vi "plcHMI_rev4.vi"() -> ()   [LabVIEW 2020]
doc: "ADS continuos synchronous write example using base blocks. \n\nThe client writes data synchronously and does wait for the respose from server."
uses:
  Agilent/AgilentTotalCluster.ctl
  Agilent/AgilentControl.ctl
  Agilent/Channel Config.ctl
  <vilib>/Platform/TimedLoop/XDataNode/timing_clust.ctl
  <vilib>/Platform/TimedLoop/XDataNode/nitl_modes.ctl
  <vilib>/Platform/TimedLoop/XDataNode/wakeup.ctl
  <userlib>/Beckhoff-LabVIEW-Interface/_DependsOn/With TypeResolving/Write Sync Single TypeResolved.vi
  <userlib>/Beckhoff-LabVIEW-Interface/_DependsOn/With TypeResolving/Read Sync Single TypeResolved.vi
  <vilib>/Platform/TimedLoop/XDataNode/XDataNode.xnode
  <vilib>/Platform/TimedLoop/XDataNode/XDNodeRunTimeDep.lvlib
panel:
  in  "Tab Control":T1(tab)
  out "error out":errorcluster
  in  "Symbol file path - MUST BE ENTERED\nLoad \"ADS Write AND Read Symbols REV X.X.xml\"":path
  out "bHasMached":bool
  out "Write Status":bool
  out "Read Status":bool
  in  "EXIT HMI":bool caption="STOP HMI\nEXIT HMI"
  out "Internal TwinCAT Handle ID Maps":dbl format="%#_12g"
  in  "802L TDK PSU Voltage Rating (abs(Volts))":i32=12000 min=1 max=50000
  in  "802L TDL PSU Peak Power (J/s)":i32=9000 min=1 max=50000
  in  "HVPS Model":u16(ring) items=["802L-12kV,9000J/s", "802L+50kV,9000J/s", "Other"]
  out "Test Interval Fault":bool
  in  "Cycle Time (Sec)":i32=15 min=0
  in  "Voltage Held by PSU":bool
  in  "Log Capacitor Voltage":bool
  in  "Log Temperature Data":bool
  out "Time Since Last Shot":string caption="Elapsed Time Text"
  in  "Duty Cycle":dbl
  in  "Current Control":bool
  out "Expected Voltage":i16
  in  "Dump":bool
  out "EOC":bool
  out "Maximum Test Number Reached":bool
  out "SCR Ready":bool
  in  "START":bool
  in  "STOP":bool
  in  "Hold":bool
  in  "Charge":bool
  in  "Shot":bool
  in  "HV Switch Mode":bool
  in  "CLEAR FAULT":bool
  in  "Manual/Auto":bool=TRUE
  out "Test Interval (Sec)":i32=15 min=0
  in  "Capacitance (uF)":sgl=1e-13 min=0 max=10000 format="%#_6f"
  in  "Target Charge Volt (V) - Min 1500V - TEMPORARY LIMIT 12kV":i32 min=-12000 max=12000 step=1
  out "Estimated Charge Time (seconds)":sgl
  in  "Hold Time Before Shot (seconds)":sgl max=1000
  in  "Max Number of Shots (Test intervals)":i16=1 min=1
  out "Shot Number":i16
  out "Charge Fault":bool=TRUE
  out "Discharge Fault":bool=TRUE
  out "Hold Fault":bool=TRUE
  out "Cap 1 Temp\nExceeded Fault":bool=TRUE
  out "Ambient Temp\nExceeded Fault":bool=TRUE
  out "PSU Fault":bool=TRUE
  out "Control Sys Fault":bool=TRUE
  out "test Running":bool
  out "Test State":string
  out "Cap 1 Voltage":i16
  out "Cap 1 Temperature":i16
  in  "Capacitor Voltage Data Log File Path (.xlsx)":path
  out "Load Temperature":i16
  out "Soft Dump Temp":i16
  out "Ambient Temp":i16
  out "Waveform Chart - Capacitor Voltage (Probe, abs(Volts))":dbl(graph)
  in  "Manual Charge Time (seconds)":sgl max=90
  in  "Reset Test Number":bool
  in  "Cap 1 Fault Temp (Cel)":i16 min=0 max=125
  in  "Capacitor Temperature Data Log File Path (.xlsx)":path
  out "Cap 1 Voltage (HVPS)":i16
  out "Capacitor Voltage":cluster{dbl, dbl}(graph)
  out "EOC":i16(graph)
  out "Soft Exception":bool
  out "PSU HV FB Fault":bool
  out "Charge FB Fault":bool
  out "Softdump FB Fault":bool
  out "SCR FB":i16(graph)
  in  "CH4 Vertical Units":string(combo)="V"
  in  "CH4 Vertical Units/div":dbl=2.0
  in  "Toggle Scope Scale":bool
  in  "CH1 Vertical Units/div":dbl=2.0
  in  "CH1 Vertical Units":string(combo)="V"
  in  "Horizontal Units":enum16{"us", "ms", "s"}(ring)
  in  "Horizontal Units/div":dbl=200.0
  out "Download":bool
  in  "Single":bool
  in  "Stop":bool
  out "Scope Trig":bool
  in  "Agilent Array":T2[](array[typedef])
  out "Process Step":u8
  out "Stop Loops":bool
  # "CONFIGURATION"
  # "Press STOP HMI instead of\nLabView Abort Execution"
  # "PSU V Rating, Peak Power\nactive when OTHER\nis selected"
  # "INPUT VARIABLES - For TDK Lambda 802L\nMust be written to before START"
  # "FAULT STATUSES"
  # "Set to -1 for automated\nfull charge to setpoint"
  # "MANUAL CONTROLS"
  # "Does not record during \"wait\" and appends to data file. Must be named with .xlsx"
  # "HV Switch Configuration"
  # "Records during \"Test Running.\" Must be named with .xlsx"
  # "Control Sys Faults"
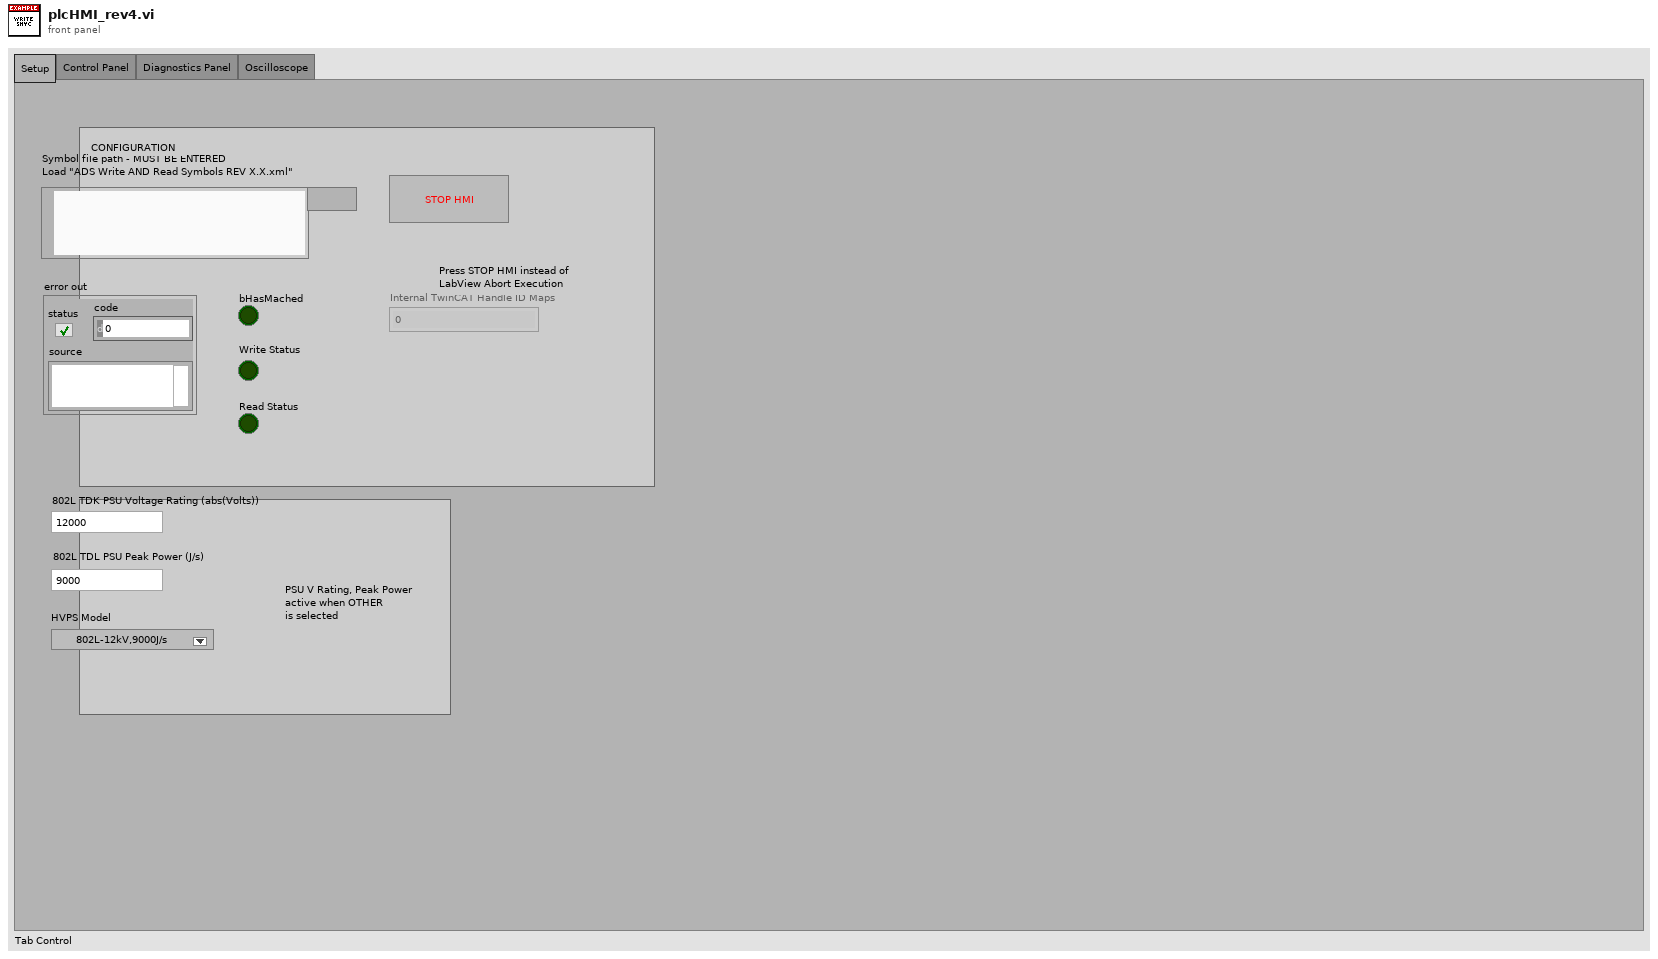
[diagram p1: front panel]
types:
  T1 = enum32{"Setup", "Control Panel", "Diagnostics Panel", "Oscilloscope"}
  T2 = typedef "AgilentTotalCluster.ctl" = cluster{"Agilent Graph":waveform(dbl)[], "Agilent Control":T3, "Agilent Setup Error":errorcluster, "Agilent Present":bool, "Enabled":bool}
  T3 = typedef "AgilentControl.ctl" = cluster{"Trig?":bool, "VISA session":refnum<visa-resource-name>, "Setup to Load":string, "Timeout (ms)":u32, "Desired Samp":enum32{"100", "250", "500", "1000", "2000", "5000", "10000", "20000", "50000", "100000", "200000", "500000", "1000000", "2000000", "4000000", "8000000"}, "Captured Samp":i32, "Desired Channels":T4[]}
  T4 = typedef "Channel Config.ctl" = cluster{"Chan Index":enum16{"Channel1", "Channel2", "Channel3", "Channel4", "MATH"}, "Name":string, "Samples":i32}
  T5 = typedef "XDNodeRunTimeDep.lvlib/timing_clust.ctl" = cluster{"Expected End [f-1]":u64, "Actual End [f-1]":u64, "Finished Late? [f-1]":bool, "Expected End [i-1]":u64, "Actual End [i-1]":u64, "Finished Late? [i-1]":bool, "Expected Start [i]":u64, "Actual Start [i]":u64, "Expected Start [f]":u64, "Actual Start [f]":u64, "Source Name":string, "Structure Name":string, "Period":i64, "Deadline":i64, "Offset":i64, "Start":i64, "Priority":i32, "Timeout":i32, "Mode":T6, "Wakeup Reason":T7, "Error":errorcluster, "Source Type":string, "Secondary Source Type":string, "Global End Time":u64, "Global Start Time":u64, "Frame Duration":u64, "Iteration Duration":u64, "Assigned CPU":i32, "I/O Scan Engine Mode":u32}
  T6 = typedef "XDNodeRunTimeDep.lvlib/nitl_modes.ctl" = enum32{"No Change", "Process missed periods, maintain original phase", "Discard missed periods, maintain original phase", "Process missed periods, ignore original phase", "Discard missed periods, ignore original phase"}
  T7 = typedef "XDNodeRunTimeDep.lvlib/wakeup.ctl" = enum32{"Normal", "Aborted", "Asynchronous wakeup", "Timing source error", "Timed loop error", "Timeout"}
  T8 = cluster{"Agilent Array[0]":T2, "Agilent Array[1]":T2, "Agilent Array[2]":T2, "Agilent Array[3]":T2, "Agilent Array[4]":T2, "Agilent Array[5]":T2, "Agilent Array[6]":T2, "Agilent Array[7]":T2, "Agilent Array[8]":T2}
  T9 = enum32{"100", "250", "500", "1000", "2000", "5000", "10000", "20000", "50000", "100000", "200000", "500000", "1000000", "2000000", "4000000", "8000000"}
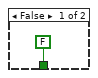
[diagram p2: hidden frame]
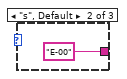
[diagram p5: hidden frame]
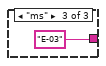
[diagram p6: hidden frame]
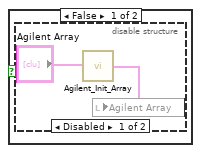
[diagram p7: hidden frame]
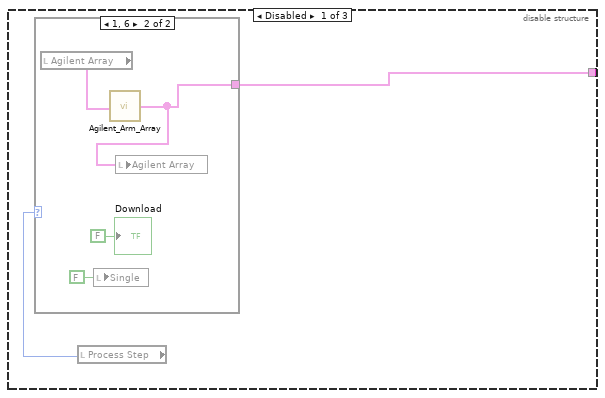
[diagram p11: hidden frame]
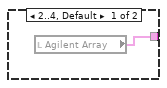
[diagram p12: hidden frame]
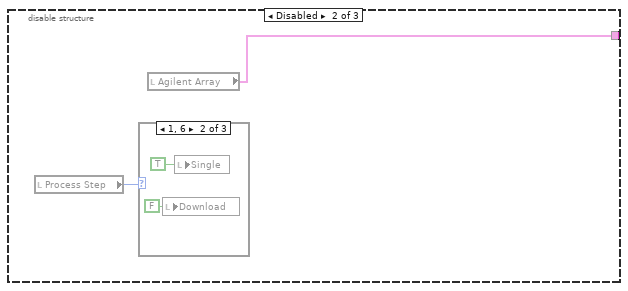
[diagram p13: hidden frame]
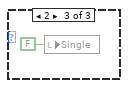
[diagram p15: hidden frame]
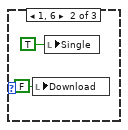
[diagram p17: hidden frame]
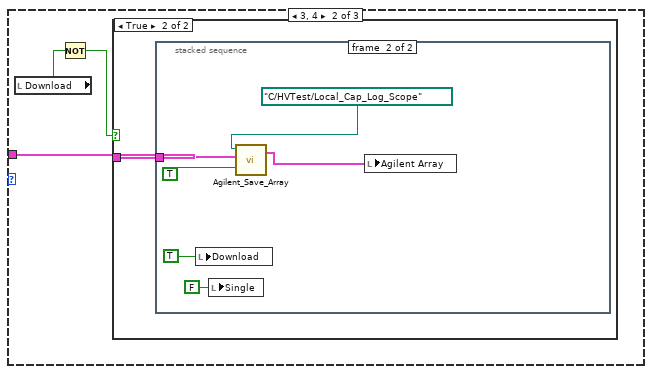
[diagram p19: hidden frame]
diagram:
  w88 = u16 17 items=["SyncLatest"=17, "AsyncLatest"=33] ("WriterMode")
  w158 = u16 33 items=["SyncLatest"=17, "AsyncLatest"=33] ("WriterMode")
  w198 = u16 33 items=["SyncLatest"=17, "AsyncLatest"=33] ("WriterMode")
  w217 = u16 33 items=["SyncLatest"=17, "AsyncLatest"=33] ("WriterMode")
  w236 = u16 33 items=["SyncLatest"=17, "AsyncLatest"=33] ("WriterMode")
  w255 = u16 33 items=["SyncLatest"=17, "AsyncLatest"=33] ("WriterMode")
  w274 = u16 33 items=["SyncLatest"=17, "AsyncLatest"=33] ("WriterMode")
  w293 = u16 17 items=["SyncLatest"=17, "AsyncLatest"=33] ("WriterMode")
  w312 = u16 17 items=["SyncLatest"=17, "AsyncLatest"=33] ("WriterMode")
  w331 = u16 17 items=["SyncLatest"=17, "AsyncLatest"=33] ("WriterMode")
  w350 = u16 17 items=["SyncLatest"=17, "AsyncLatest"=33] ("WriterMode")
  w369 = u16 17 items=["SyncLatest"=17, "AsyncLatest"=33] ("WriterMode")
  w388 = u16 17 items=["SyncLatest"=17, "AsyncLatest"=33] ("WriterMode")
  w407 = u16 17 items=["SyncLatest"=17, "AsyncLatest"=33] ("WriterMode")
  w422 = u16 17 items=["SyncLatest"=17, "AsyncLatest"=33] ("WriterMode")
  # "Variables/ Control"
  # "Documentation:\nCode separated vertically into two main sections - Write and read\nThey are further separated into BOOL and numeric\nThe OR gates wire all the error lines and the EXIT HMI button to a WHILE LOOP STOP\nThere current delay time on the routine is 100ms\nAll the AND gates connect the typecast resolve lines to the bHasMatched indicator\nThe second and third set of AND gates connect the write statuses to the Write Status indicator\nThe same is done for the read status indicator"
  # "WRITE NUMERICS"
  # "WRITE BOOLS"
  # "Select Symbol N"
  # "Read Initialization"
  # "Release \nTypeResolver"
  # "Release Writer"
  # "Send Request"
  # "Init \nTypeResolver"
  # "Init Writer"
  # "Select Symbol"
  # "Initialization"
  # "Call Release handle block\nat the end, when all nodes\nhave finished their execution"
  # "There must be only one release\nafter every init block.\nRelease block must be called\nalways at the end."
  # "Release"
  # "Symbol Interface"
  n1 = disable-structure shown="Enabled" {
    disable-tunnel: [w428 _] -> w426
    disable-tunnel: [w427 w430] -> w425
    frame Disabled {
      # "Using Symbol Interface"
      n2 = call <userlib>:"Symbol Interface.vi"() -> ("PortInfo"=w427:string, "error out"=w428:errorcluster)  [unwired: 14 in]
    }
    frame Enabled {
      # "Using Symbol File"
      n3 = Path To String(path="Symbol file path - MUST BE ENTERED\nLoad \"ADS Write AND Read Symbols REV X.X.xml\"") -> (string=w430:string)
    }
  }
  n4 = call <userlib>:"Init.vi"("XMLDescription"=w425, "error in (no error)"=w426) -> ("Handle"=w38:u32, "ReadGrpSymbols"=w20:string[], "WriteGrpSymbols"=w26:string[], "error out"=w2:errorcluster)  [unwired: 9 in, 1 out]
  n5 = Index Array(array=w26, index=0) -> (element=w13:string)
  n6 = Index Array(array=w26, index=21) -> (element=w25:string)
  n7 = Index Array(array=w26, index=20) -> (element=w31:string)
  n8 = Index Array(array=w26, index=14) -> (element=w3:string)
  n9 = Index Array(array=w26, index=9) -> (element=w275:string)
  n10 = Index Array(array=w26, index=10) -> (element=w256:string)
  n11 = Index Array(array=w26, index=12) -> (element=w218:string)
  n12 = Index Array(array=w26, index=11) -> (element=w237:string)
  n13 = Index Array(array=w26, index=13) -> (element=w199:string)
  n14 = Index Array(array=w26, index=18) -> (element=w39:string)
  n15 = Index Array(array=w26, index=19) -> (element=w32:string)
  n16 = Index Array(array=w26, index=7) -> (element=w294:string)
  n17 = Index Array(array=w26, index=2) -> (element=w389:string)
  n18 = Index Array(array=w26, index=3) -> (element=w370:string)
  n19 = Index Array(array=w26, index=5) -> (element=w332:string)
  n20 = Index Array(array=w26, index=4) -> (element=w351:string)
  n21 = Index Array(array=w26, index=6) -> (element=w313:string)
  n22 = Index Array(array=w26, index=1) -> (element=w408:string)
  n23 = Index Array(array=w26, index=16) -> (element=w6:string)
  n24 = Index Array(array=w26, index=8) -> (element=w87:string)
  n25 = Index Array(array=w26, index=15) -> (element=w159:string)
  n26 = Index Array(array=w26, index=17) -> (element=w8:string)
  n27 = call <userlib>:"Init Writer.vi"("Handle"=w38, "SymbolName"=w275, "WriterMode"=w274, "error constant"=w2) -> ("Handle"=w270:u32, "SymbolName"=w269:string, "WriterMode"=w268:u16, "WriteHandle"=w266:u32, "error IO"=w267:errorcluster)  [unwired: 7 in]
  n28 = call <userlib>:"Init Writer.vi"("Handle"=w38, "SymbolName"=w256, "WriterMode"=w255, "error constant"=w2) -> ("Handle"=w254:u32, "SymbolName"=w253:string, "WriterMode"=w252:u16, "WriteHandle"=w251:u32, "error IO"=w250:errorcluster)  [unwired: 7 in]
  n29 = call <userlib>:"Init Writer.vi"("Handle"=w38, "SymbolName"=w218, "WriterMode"=w217, "error constant"=w2) -> ("Handle"=w216:u32, "SymbolName"=w215:string, "WriterMode"=w214:u16, "WriteHandle"=w213:u32, "error IO"=w212:errorcluster)  [unwired: 7 in]
  n30 = call <userlib>:"Init Type.vi"("Handle"=w38, "SymbolName"=w275, "error in"=w2) -> ("Handle"=w259:u32, "TypeHdl"=w258:u32, "error IO"=w257:errorcluster)  [unwired: 7 in, 3 out]
  n31 = call <userlib>:"Init Type.vi"("Handle"=w38, "SymbolName"=w256, "error in"=w2) -> ("Handle"=w249:u32, "TypeHdl"=w248:u32, "error IO"=w247:errorcluster)  [unwired: 7 in, 3 out]
  n32 = call <userlib>:"Init Writer.vi"("Handle"=w38, "SymbolName"=w237, "WriterMode"=w236, "error constant"=w2) -> ("Handle"=w235:u32, "SymbolName"=w234:string, "WriterMode"=w233:u16, "WriteHandle"=w232:u32, "error IO"=w231:errorcluster)  [unwired: 7 in]
  n33 = call <userlib>:"Init Type.vi"("Handle"=w38, "SymbolName"=w218, "error in"=w2) -> ("Handle"=w211:u32, "TypeHdl"=w210:u32, "error IO"=w209:errorcluster)  [unwired: 7 in, 3 out]
  n34 = call <userlib>:"Init Writer.vi"("Handle"=w38, "SymbolName"=w199, "WriterMode"=w198, "error constant"=w2) -> ("Handle"=w197:u32, "SymbolName"=w196:string, "WriterMode"=w195:u16, "WriteHandle"=w194:u32, "error IO"=w193:errorcluster)  [unwired: 7 in]
  n35 = call <userlib>:"Init Type.vi"("Handle"=w38, "SymbolName"=w237, "error in"=w2) -> ("Handle"=w230:u32, "TypeHdl"=w229:u32, "error IO"=w228:errorcluster)  [unwired: 7 in, 3 out]
  n36 = call <userlib>:"Init Type.vi"("Handle"=w38, "SymbolName"=w199, "error in"=w2) -> ("Handle"=w192:u32, "TypeHdl"=w191:u32, "error IO"=w190:errorcluster)  [unwired: 7 in, 3 out]
  n37 = call <userlib>:"Init Writer.vi"("Handle"=w38, "SymbolName"=w294, "WriterMode"=w293, "error constant"=w2) -> ("Handle"=w292:u32, "SymbolName"=w291:string, "WriterMode"=w290:u16, "WriteHandle"=w289:u32, "error IO"=w288:errorcluster)  [unwired: 7 in]
  n38 = call <userlib>:"Init Writer.vi"("Handle"=w38, "SymbolName"=w389, "WriterMode"=w388, "error constant"=w2) -> ("Handle"=w384:u32, "SymbolName"=w383:string, "WriterMode"=w382:u16, "WriteHandle"=w380:u32, "error IO"=w381:errorcluster)  [unwired: 7 in]
  n39 = call <userlib>:"Init Writer.vi"("Handle"=w38, "SymbolName"=w370, "WriterMode"=w369, "error constant"=w2) -> ("Handle"=w368:u32, "SymbolName"=w367:string, "WriterMode"=w366:u16, "WriteHandle"=w365:u32, "error IO"=w364:errorcluster)  [unwired: 7 in]
  n40 = call <userlib>:"Init Writer.vi"("Handle"=w38, "SymbolName"=w332, "WriterMode"=w331, "error constant"=w2) -> ("Handle"=w330:u32, "SymbolName"=w329:string, "WriterMode"=w328:u16, "WriteHandle"=w327:u32, "error IO"=w326:errorcluster)  [unwired: 7 in]
  n41 = call <userlib>:"Init Type.vi"("Handle"=w38, "SymbolName"=w294, "error in"=w2) -> ("Handle"=w287:u32, "TypeHdl"=w286:u32, "error IO"=w285:errorcluster)  [unwired: 7 in, 3 out]
  n42 = call <userlib>:"Init Type.vi"("Handle"=w38, "SymbolName"=w389, "error in"=w2) -> ("Handle"=w373:u32, "TypeHdl"=w372:u32, "error IO"=w371:errorcluster)  [unwired: 7 in, 3 out]
  n43 = call <userlib>:"Init Type.vi"("Handle"=w38, "SymbolName"=w370, "error in"=w2) -> ("Handle"=w363:u32, "TypeHdl"=w362:u32, "error IO"=w361:errorcluster)  [unwired: 7 in, 3 out]
  n44 = call <userlib>:"Init Writer.vi"("Handle"=w38, "SymbolName"=w351, "WriterMode"=w350, "error constant"=w2) -> ("Handle"=w349:u32, "SymbolName"=w348:string, "WriterMode"=w347:u16, "WriteHandle"=w346:u32, "error IO"=w345:errorcluster)  [unwired: 7 in]
  n45 = call <userlib>:"Init Type.vi"("Handle"=w38, "SymbolName"=w332, "error in"=w2) -> ("Handle"=w325:u32, "TypeHdl"=w324:u32, "error IO"=w323:errorcluster)  [unwired: 7 in, 3 out]
  n46 = call <userlib>:"Init Writer.vi"("Handle"=w38, "SymbolName"=w313, "WriterMode"=w312, "error constant"=w2) -> ("Handle"=w311:u32, "SymbolName"=w310:string, "WriterMode"=w309:u16, "WriteHandle"=w308:u32, "error IO"=w307:errorcluster)  [unwired: 7 in]
  n47 = call <userlib>:"Init Type.vi"("Handle"=w38, "SymbolName"=w351, "error in"=w2) -> ("Handle"=w344:u32, "TypeHdl"=w343:u32, "error IO"=w342:errorcluster)  [unwired: 7 in, 3 out]
  n48 = call <userlib>:"Init Type.vi"("Handle"=w38, "SymbolName"=w313, "error in"=w2) -> ("Handle"=w306:u32, "TypeHdl"=w305:u32, "error IO"=w304:errorcluster)  [unwired: 7 in, 3 out]
  n49 = call <userlib>:"Init Writer.vi"("Handle"=w38, "SymbolName"=w408, "WriterMode"=w407, "error constant"=w2) -> ("Handle"=w406:u32, "SymbolName"=w405:string, "WriterMode"=w404:u16, "WriteHandle"=w403:u32, "error IO"=w402:errorcluster)  [unwired: 7 in]
  n50 = call <userlib>:"Init Type.vi"("Handle"=w38, "SymbolName"=w408, "error in"=w2) -> ("Handle"=w401:u32, "TypeHdl"=w400:u32, "error IO"=w399:errorcluster)  [unwired: 7 in, 3 out]
  n51 = call <userlib>:"Init Writer.vi"("Handle"=w38, "SymbolName"=w13, "WriterMode"=w422, "error constant"=w2) -> ("Handle"=w421:u32, "SymbolName"=w420:string, "WriterMode"=w419:u16, "WriteHandle"=w418:u32, "error IO"=w417:errorcluster)  [unwired: 7 in]
  n52 = call <userlib>:"Init Type.vi"("Handle"=w38, "SymbolName"=w13, "error in"=w2) -> ("Handle"=w416:u32, "TypeHdl"=w415:u32, "error IO"=w410:errorcluster)  [unwired: 7 in, 3 out]
  n53 = call <userlib>:"Init Writer.vi"("Handle"=w38, "SymbolName"=w159, "WriterMode"=w158, "error constant"=w2) -> ("Handle"=w154:u32, "SymbolName"=w153:string, "WriterMode"=w152:u16, "WriteHandle"=w144:u32, "error IO"=w151:errorcluster)  [unwired: 7 in]
  n54 = call <userlib>:"Init Type.vi"("Handle"=w38, "SymbolName"=w159, "error in"=w2) -> ("Handle"=w149:u32, "TypeHdl"=w147:u32, "error IO"=w148:errorcluster)  [unwired: 7 in, 3 out]
  n55 = Index Array(array=w20, index=2) -> (element=w140:string)
  n56 = Index Array(array=w20, index=4) -> (element=w136:string)
  n57 = call <userlib>:"Init Writer.vi"("Handle"=w38, "SymbolName"=w87, "WriterMode"=w88, "error constant"=w2) -> ("Handle"=w86:u32, "SymbolName"=w85:string, "WriterMode"=w84:u16, "WriteHandle"=w83:u32, "error IO"=w82:errorcluster)  [unwired: 7 in]
  n58 = Index Array(array=w20, index=1) -> (element=w176:string)
  n59 = Index Array(array=w20, index=21) -> (element=w53:string)
  n60 = Index Array(array=w20, index=22) -> (element=w50:string)
  n61 = call <userlib>:"Init Type.vi"("Handle"=w38, "SymbolName"=w87, "error in"=w2) -> ("Handle"=w81:u32, "TypeHdl"=w80:u32, "error IO"=w79:errorcluster)  [unwired: 7 in, 3 out]
  n62 = Index Array(array=w20, index=0) -> (element=w175:string)
  n63 = Index Array(array=w20, index=3) -> (element=w137:string)
  n64 = Index Array(array=w20, index=20) -> (element=w58:string)
  n65 = Index Array(array=w20, index=23) -> (element=w49:string)
  n66 = Index Array(array=w20, index=16) -> (element=w142:string)
  n67 = Index Array(array=w20, index=24) -> (element=w47:string)
  n68 = Index Array(array=w20, index=11) -> (element=w164:string)
  n69 = Index Array(array=w20, index=10) -> (element=w165:string)
  n70 = Index Array(array=w20, index=17) -> (element=w61:string)
  n71 = Index Array(array=w20, index=18) -> (element=w60:string)
  n72 = Index Array(array=w20, index=13) -> (element=w162:string)
  n73 = Index Array(array=w20, index=27) -> (element=w18:string)
  n74 = Index Array(array=w20, index=12) -> (element=w163:string)
  n75 = Index Array(array=w20, index=15) -> (element=w160:string)
  n76 = Index Array(array=w20, index=19) -> (element=w59:string)
  n77 = Index Array(array=w20, index=26) -> (element=w19:string)
  n78 = Index Array(array=w20, index=5) -> (element=w72:string)
  n79 = Index Array(array=w20, index=6) -> (element=w130:string)
  n80 = Index Array(array=w20, index=9) -> (element=w174:string)
  n81 = Index Array(array=w20, index=14) -> (element=w161:string)
  n82 = Index Array(array=w20, index=8) -> (element=w132:string)
  n83 = Index Array(array=w20, index=25) -> (element=w36:string)
  n84 = Index Array(array=w20, index=7) -> (element=w131:string)
  n85 = node-c288(i64 10 ("Period")) -> (w96:T5)  [unwired: 2 in]
  n86 = timed-loop {
    tunnel: w421 -> [w733]
    tunnel: w420 -> [w732]
    tunnel: w419 -> [w731]
    tunnel: w418 -> [w730]
    tunnel: w416 -> [w975]
    tunnel: w415 -> [w974]
    tunnel: [w728] -> w414
    tunnel: [w727] -> w413
    tunnel: [w973] -> w412
    tunnel: [w972] -> w411
    tunnel: w406 -> [w970]
    tunnel: w405 -> [w969]
    tunnel: w404 -> [w968]
    tunnel: w403 -> [w967]
    tunnel: w401 -> [w965]
    tunnel: w400 -> [w964]
    tunnel: [w962] -> w397
    tunnel: [w961] -> w396
    tunnel: [w960] -> w394
    tunnel: [w959] -> w393
    tunnel: w384 -> [w958]
    tunnel: w383 -> [w957]
    tunnel: w382 -> [w956]
    tunnel: w380 -> [w954]
    tunnel: [w953] -> w379
    tunnel: [w952] -> w378
    tunnel: [w951] -> w375
    tunnel: [w950] -> w374
    tunnel: w373 -> [w949]
    tunnel: w372 -> [w948]
    tunnel: w368 -> [w946]
    tunnel: w367 -> [w945]
    tunnel: w366 -> [w944]
    tunnel: w365 -> [w943]
    tunnel: w363 -> [w941]
    tunnel: w362 -> [w940]
    tunnel: [w938] -> w359
    tunnel: [w937] -> w358
    tunnel: [w936] -> w356
    tunnel: [w935] -> w355
    tunnel: w349 -> [w934]
    tunnel: w348 -> [w933]
    tunnel: w347 -> [w932]
    tunnel: w346 -> [w931]
    tunnel: w344 -> [w929]
    tunnel: w343 -> [w928]
    tunnel: [w926] -> w340
    tunnel: [w925] -> w339
    tunnel: [w924] -> w337
    tunnel: [w923] -> w336
    tunnel: w330 -> [w922]
    tunnel: w329 -> [w921]
    tunnel: w328 -> [w920]
    tunnel: w327 -> [w919]
    tunnel: w325 -> [w917]
    tunnel: w324 -> [w916]
    tunnel: [w914] -> w321
    tunnel: [w913] -> w320
    tunnel: [w912] -> w318
    tunnel: [w911] -> w317
    tunnel: w311 -> [w910]
    tunnel: w310 -> [w909]
    tunnel: w309 -> [w908]
    tunnel: w308 -> [w907]
    tunnel: w306 -> [w905]
    tunnel: w305 -> [w904]
    tunnel: [w902] -> w302
    tunnel: [w901] -> w301
    tunnel: [w900] -> w299
    tunnel: [w899] -> w298
    tunnel: w292 -> [w898]
    tunnel: w291 -> [w897]
    tunnel: w290 -> [w896]
    tunnel: w289 -> [w895]
    tunnel: w287 -> [w893]
    tunnel: w286 -> [w892]
    tunnel: [w890] -> w283
    tunnel: [w889] -> w282
    tunnel: [w888] -> w280
    tunnel: [w887] -> w279
    tunnel: w270 -> [w886]
    tunnel: w269 -> [w885]
    tunnel: w268 -> [w884]
    tunnel: w266 -> [w882]
    tunnel: [w881] -> w265
    tunnel: [w880] -> w264
    tunnel: [w879] -> w261
    tunnel: [w878] -> w260
    tunnel: w259 -> [w877]
    tunnel: w258 -> [w876]
    tunnel: w254 -> [w874]
    tunnel: w253 -> [w873]
    tunnel: w252 -> [w872]
    tunnel: w251 -> [w871]
    tunnel: w249 -> [w869]
    tunnel: w248 -> [w868]
    tunnel: [w866] -> w245
    tunnel: [w865] -> w244
    tunnel: [w864] -> w242
    tunnel: [w863] -> w241
    tunnel: w235 -> [w862]
    tunnel: w234 -> [w861]
    tunnel: w233 -> [w860]
    tunnel: w232 -> [w859]
    tunnel: w230 -> [w857]
    tunnel: w229 -> [w856]
    tunnel: [w854] -> w226
    tunnel: [w853] -> w225
    tunnel: [w852] -> w223
    tunnel: [w851] -> w222
    tunnel: w216 -> [w850]
    tunnel: w215 -> [w849]
    tunnel: w214 -> [w848]
    tunnel: w213 -> [w847]
    tunnel: w211 -> [w845]
    tunnel: w210 -> [w844]
    tunnel: [w842] -> w207
    tunnel: [w841] -> w206
    tunnel: [w840] -> w204
    tunnel: [w839] -> w203
    tunnel: w197 -> [w838]
    tunnel: w196 -> [w837]
    tunnel: w195 -> [w836]
    tunnel: w194 -> [w835]
    tunnel: w192 -> [w833]
    tunnel: w191 -> [w832]
    tunnel: [w830] -> w188
    tunnel: [w829] -> w187
    tunnel: [w828] -> w185
    tunnel: [w827] -> w184
    tunnel: w176 -> [w826]
    tunnel: w175 -> [w825]
    tunnel: w174 -> [w824]
    tunnel: [w823] -> w125
    tunnel: w165 -> [w822]
    tunnel: w164 -> [w821]
    tunnel: w163 -> [w820]
    tunnel: w162 -> [w819]
    tunnel: w161 -> [w818]
    tunnel: w160 -> [w817]
    tunnel: [w816] -> w93
    tunnel: [w815] -> w124
    tunnel: [w814] -> w123
    tunnel: [w813] -> w122
    tunnel: [w812] -> w121
    tunnel: [w756] -> w120
    tunnel: [w754] -> w119
    shift-right: [w657] -> w424
    shift-left: w417 -> [w729]
    shift-right: [w656] -> w423
    shift-left: w410 -> [w971]
    shift-right: [w654] -> w395
    shift-left: w402 -> [w966]
    shift-right: [w653] -> w392
    shift-left: w399 -> [w963]
    shift-right: [w651] -> w377
    shift-left: w381 -> [w955]
    shift-right: [w650] -> w376
    shift-left: w371 -> [w947]
    shift-right: [w648] -> w357
    shift-left: w364 -> [w942]
    shift-right: [w647] -> w354
    shift-left: w361 -> [w939]
    shift-right: [w645] -> w338
    shift-left: w345 -> [w930]
    shift-right: [w644] -> w335
    shift-left: w342 -> [w927]
    shift-right: [w642] -> w319
    shift-left: w326 -> [w918]
    shift-right: [w641] -> w316
    shift-left: w323 -> [w915]
    shift-right: [w639] -> w300
    shift-left: w307 -> [w906]
    shift-right: [w638] -> w297
    shift-left: w304 -> [w903]
    shift-right: [w636] -> w281
    shift-left: w288 -> [w894]
    shift-right: [w635] -> w278
    shift-left: w285 -> [w891]
    shift-right: [w634] -> w263
    shift-left: w267 -> [w883]
    shift-right: [w633] -> w262
    shift-left: w257 -> [w875]
    shift-right: [w631] -> w243
    shift-left: w250 -> [w870]
    shift-right: [w630] -> w240
    shift-left: w247 -> [w867]
    shift-right: [w628] -> w224
    shift-left: w231 -> [w858]
    shift-right: [w627] -> w221
    shift-left: w228 -> [w855]
    shift-right: [w625] -> w205
    shift-left: w212 -> [w846]
    shift-right: [w624] -> w202
    shift-left: w209 -> [w843]
    shift-right: [w622] -> w186
    shift-left: w193 -> [w834]
    shift-right: [w621] -> w183
    shift-left: w190 -> [w831]
    tunnel: w154 -> [w796]
    tunnel: w153 -> [w795]
    tunnel: w152 -> [w794]
    tunnel: [w792] -> w12
    tunnel: [w791] -> w150
    tunnel: w149 -> [w790]
    tunnel: w147 -> [w788]
    tunnel: [w787] -> w146
    tunnel: [w786] -> w145
    tunnel: w144 -> [w785]
    tunnel: w142 -> [w784]
    tunnel: [w755] -> w118
    tunnel: [w778] -> w127
    tunnel: w2 -> [w777]
    tunnel: [w775] -> w126
    tunnel: w140 -> [w774]
    tunnel: w137 -> [w770]
    tunnel: w136 -> [w769]
    tunnel: [w760] -> w128
    tunnel: [w759] -> w129
    tunnel: w132 -> [w753]
    tunnel: w131 -> [w752]
    tunnel: w130 -> [w751]
    tunnel: [w738] -> w69
    tunnel: [w737] -> w68
    tunnel: [w736] -> w67
    timing: w96 -> [_]
    timing-out: [_] -> w95
    tunnel: w38 -> [w726]
    tunnel: [w619] -> w71
    tunnel: w86 -> [w614]
    tunnel: w85 -> [w613]
    tunnel: w84 -> [w612]
    tunnel: w83 -> [w611]
    tunnel: w81 -> [w609]
    tunnel: w80 -> [w608]
    tunnel: [w605] -> w78
    tunnel: [w604] -> w77
    tunnel: [w603] -> w76
    tunnel: [w602] -> w75
    tunnel: [w595] -> w70
    tunnel: w72 -> [w591]
    tunnel: [w590] -> w66
    tunnel: w61 -> [w586]
    tunnel: w60 -> [w581]
    tunnel: w59 -> [w580]
    tunnel: w58 -> [w579]
    tunnel: [w576] -> w57
    tunnel: [w574] -> w56
    tunnel: [w569] -> w55
    tunnel: [w568] -> w42
    tunnel: w53 -> [w566]
    tunnel: w50 -> [w541]
    tunnel: w49 -> [w540]
    tunnel: w47 -> [w533]
    tunnel: [w529] -> w46
    tunnel: [w528] -> w45
    tunnel: [w527] -> w44
    tunnel: [w526] -> w43
    tunnel: w39 -> [w525]
    tunnel: w38 -> [w438]
    tunnel: w2 -> [w524]
    tunnel: [w521] -> w30
    tunnel: [w520] -> _
    tunnel: w36 -> [w516]
    tunnel: [w512] -> w35
    tunnel: w32 -> [w511]
    tunnel: w31 -> [w510]
    tunnel: w2 -> [w487]
    tunnel: [w505] -> w29
    tunnel: [w504] -> w28
    tunnel: w25 -> [w491]
    tunnel: [w486] -> w24
    tunnel: w19 -> [w473]
    tunnel: w18 -> [w472]
    tunnel: [w467] -> w17
    tunnel: [w466] -> w16
    shift-right: [w464] -> w15
    shift-left: w151 -> [w793]
    shift-right: [w463] -> w14
    shift-left: w148 -> [w789]
    tunnel: w2 -> [w456]
    tunnel: [w453] -> w7
    shift-right: [w461] -> w10
    shift-left: w82 -> [w610]
    shift-right: [w460] -> w9
    shift-left: w79 -> [w607]
    tunnel: w8 -> [w455]
    tunnel: w6 -> [w448]
    tunnel: w2 -> [w447]
    tunnel: [w446] -> w5
    tunnel: w3 -> [w439]
    tunnel: w2 -> [w437]
    tunnel: [w436] -> w1
    stop <- w431 stop-if-true
    # "Stop Loop on Error (OR gates)"
    # "Error Stop Loop AND"
    # "Typecast Match AND"
    # "Write Status AND"
    # "READ BOOLS"
    # "READ NUMERICS"
    # "STOP HMI via error or EXIT button"
    # "Check Read status and\nthen convert Variant \nto LabVIEW type (AND gates)"
    # "Sync Read Single"
    n87 = node-c288() -> (w620:errorcluster)  [unwired: 1 in]
    n88 = disable-structure shown="Enabled" {
      frame Enabled {
        n89 = flat-sequence {
          tunnel: [w1111] -> w1055
          tunnel: w1055 -> [w1130]
          frame #0 {
            n90 = disable-structure shown="Enabled" {
              frame Enabled {
                n91 = feedback #1(TRUE) -> (w1057:bool)
                n92 = And(x=TRUE, y=w1057) -> (x .and. y?=w1060:bool)
                n93 = case shown="True" w1060 {
                  tunnel: [FALSE FALSE] -> w1058
                  frame False {
                  }
                  frame True {
                    n94 = local read "Agilent Array"() -> (w1063:T2[])
                    n95 = call "Agilent_Init_Array.vi"("Agilent Array In"=w1063) -> ("Agilent Array Out"=w1064:T2[])
                    n96 = call "Agilent_Arm_Array.vi"("Agilent Array In"=w1064) -> ("Agilent Array Out"=w1062:T2[])
                    n97 = local write "Agilent Array"(w1062) -> ()
                  }
                }
                n98 = feedback-in #1(w1058) -> ()
              }
              frame Disabled {
              }
            }
          }
          frame #1 {
            n99 = case shown="True" "Toggle Scope Scale" {
              frame False {
              }
              frame True {
                n100 = Number To Decimal String(number="CH4 Vertical Units/div") -> (decimal integer string=w1070:string)  [unwired: 1 in]
                n101 = Number To Decimal String(number="Horizontal Units/div") -> (decimal integer string=w1078:string)  [unwired: 1 in]
                n102 = Number To Decimal String(number="CH1 Vertical Units/div") -> (decimal integer string=w1076:string)  [unwired: 1 in]
                n103 = case shown="\"us\"" "Horizontal Units" {
                  tunnel: ["E-06" "E-00" "E-03"] -> w1087
                  frame "us" {
                  }
                  frame "s", Default {
                  }
                  frame "ms" {
                  }
                }
                n104 = Concatenate Strings(":CHAN4:SCAL " ("write buffer"), w1070, "CH4 Vertical Units") -> (w1069:string)
                n105 = Concatenate Strings(":CHAN1:SCAL " ("write buffer"), w1076, "CH1 Vertical Units") -> (w1083:string)
                n106 = Concatenate Strings(":TIM:SCAL " ("write buffer"), w1078, w1087) -> (w1086:string)
                n107 = VISA Open(VISA resource name=refnum<visa-resource-name> "HV_Test_Scope") -> (VISA resource name=w1081:refnum<visa-resource-name>, error out=w1082:errorcluster)  [unwired: 4 in]
                n108 = VISA Write(VISA resource name=w1081, write buffer=w1086, error in (no error)=w1082) -> (VISA resource name out=w1090:refnum<visa-resource-name>, error out=w1089:errorcluster)  [unwired: 1 out]
                n109 = VISA Write(VISA resource name=w1090, write buffer=w1083, error in (no error)=w1089) -> (VISA resource name out=w1075:refnum<visa-resource-name>, error out=w1073:errorcluster)  [unwired: 1 out]
                n110 = VISA Write(VISA resource name=w1075, write buffer=w1069, error in (no error)=w1073) -> (VISA resource name out=w1074:refnum<visa-resource-name>, error out=w1072:errorcluster)  [unwired: 1 out]
                n111 = VISA Close(VISA resource name=w1074, error in (no error)=w1072) -> ()  [unwired: 1 out]
              }
            }
          }
          frame #2 {
            n112 = disable-structure shown="Enabled" {
              frame Enabled {
                n113 = case shown="True" "Stop" {
                  frame False {
                    n114 = disable-structure shown="Disabled" {
                      frame Disabled {
                        n115 = call "Agilent_Init_Array.vi"("Agilent Array In"="Agilent Array") -> ("Agilent Array Out"=w1097:T2[])
                        n116 = local write "Agilent Array"(w1097) -> ()
                      }
                      frame Enabled {
                      }
                    }
                  }
                  frame True {
                    n117 = VISA Open(VISA resource name=refnum<visa-resource-name> "HV_Test_Scope") -> (VISA resource name=w1103:refnum<visa-resource-name>, error out=w1104:errorcluster)  [unwired: 4 in]
                    n118 = VISA Write(VISA resource name=w1103, write buffer=":STOP", error in (no error)=w1104) -> (VISA resource name out=w1101:refnum<visa-resource-name>, error out=w1102:errorcluster)  [unwired: 1 out]
                    n119 = VISA Close(VISA resource name=w1101, error in (no error)=w1102) -> ()  [unwired: 1 out]
                  }
                }
              }
              frame Disabled {
              }
            }
            n120 = case shown="True" "Single" {
              frame False {
              }
              frame True {
                n121 = VISA Open(VISA resource name=refnum<visa-resource-name> "HV_Test_Scope") -> (VISA resource name=w1109:refnum<visa-resource-name>, error out=w1110:errorcluster)  [unwired: 4 in]
                n122 = VISA Write(VISA resource name=w1109, write buffer=":SINGLE", error in (no error)=w1110) -> (VISA resource name out=w1107:refnum<visa-resource-name>, error out=w1108:errorcluster)  [unwired: 1 out]
                n123 = VISA Close(VISA resource name=w1107, error in (no error)=w1108) -> ()  [unwired: 1 out]
              }
            }
          }
          frame #3 {
            n124 = disable-structure shown="Enabled" {
              disable-tunnel: [w1113 w1120 w1125] -> w1111
              frame Disabled {
                n125 = local read "Process Step"() -> (w1112:u8)
                n126 = case shown="1, 6" w1112 {
                  tunnel: [w1114 w1118] -> w1113
                  frame 2..4, Default {
                    n127 = local read "Agilent Array"() -> (w1114:T2[])
                  }
                  frame 1, 6 {
                    n128 = local read "Agilent Array"() -> (w1115:T2[])
                    n129 = local write "Single"(FALSE ("Single")) -> ()
                    n130 = call "Agilent_Arm_Array.vi"("Agilent Array In"=w1115) -> ("Agilent Array Out"=w1118:T2[])
                    n131 = local write "Agilent Array"(w1118) -> ()
                    "Download" <- FALSE ("Downloading")
                  }
                }
              }
              frame Disabled {
                n132 = local read "Process Step"() -> (w1119:u8)
                n133 = case shown="1, 6" w1119 {
                  frame 0, Default {
                  }
                  frame 1, 6 {
                    n134 = local write "Download"(FALSE ("Download")) -> ()
                    n135 = local write "Single"(TRUE ("Single")) -> ()
                  }
                  frame 2 {
                    n136 = local write "Single"(FALSE ("Single")) -> ()
                  }
                }
                n137 = local read "Agilent Array"() -> (w1120:T2[])
              }
              frame Enabled {
                n138 = local read "Process Step"() -> (w1124:u8)
                n139 = case shown="2, 7" w1124 {
                  frame 0, Default {
                  }
                  frame 1, 6 {
                    n140 = local write "Download"(FALSE ("Download")) -> ()
                    n141 = local write "Single"(TRUE ("Single")) -> ()
                  }
                  frame 2, 7 {
                    n142 = local write "Single"(FALSE ("Single")) -> ()
                  }
                }
                n143 = local read "Agilent Array"() -> (w1125:T2[])
              }
            }
          }
          frame #4 {
            n144 = local read "Process Step"() -> (w1129:u8)
            n145 = case shown="0" w1129 {
              tunnel: w1130 -> [_ w1133 w1146]
              frame Default {
              }
              frame 3, 4 {
                n146 = local read "Download"() -> (w1132:bool)
                n147 = Not(x=w1132) -> (.not. x?=w1131:bool)
                n148 = case shown="True" w1131 {
                  tunnel: w1133 -> [_ w1134]
                  frame False {
                  }
                  frame True {
                    n149 = stacked-sequence {
                      tunnel: w1134 -> [_ w1144]
                      frame #0 {
                        n150 = local read "Agilent Array"() -> (w1138:T2[])
                        n151 = Array To Cluster(array=w1138) -> (cluster=w1137:T8)
                        n152 = Unbundle By Name(w1137) -> ("Agilent Array[0].Agilent Control.Desired Samp"=w1135:T9)
                        n153 = call "GF_SetRecordLengthProperly.vi"("Num Samples"=w1135, "VISA resource name"=refnum<visa-resource-name> "HV_Test_Scope") -> ()  [unwired: 1 in, 2 out]
                      }
                      frame #1 {
                        n154 = local write "Download"(TRUE ("Downloading")) -> ()
                        n155 = local write "Single"(FALSE ("Single")) -> ()
                        n156 = call "Agilent_Save_Array.vi"("Agilent Download"=TRUE, "Agilent Array In"=w1144, "File Path"=path "C:/HVTest/Local_Cap_Log_Scope") -> ("Agilent Array Out"=w1142:T2[])  [unwired: 1 in, 1 out]
                        n157 = local write "Agilent Array"(w1142) -> ()
                      }
                    }
                  }
                }
              }
              frame 0 {
                n158 = local read "Maximum Test Number Reached"() -> (w1145:bool)
                n159 = case shown="True" w1145 {
                  tunnel: w1146 -> [_ w1149]
                  frame False {
                  }
                  frame True {
                    n160 = local read "Download"() -> (w1148:bool)
                    n161 = Not(x=w1148) -> (.not. x?=w1147:bool)
                    n162 = case shown="True" w1147 {
                      tunnel: w1149 -> [_ w1150]
                      frame False {
                      }
                      frame True {
                        n163 = stacked-sequence {
                          tunnel: w1150 -> [_ w1160]
                          frame #0 {
                            n164 = local read "Agilent Array"() -> (w1154:T2[])
                            n165 = Array To Cluster(array=w1154) -> (cluster=w1153:T8)
                            n166 = Unbundle By Name(w1153) -> ("Agilent Array[0].Agilent Control.Desired Samp"=w1151:T9)
                            n167 = call "GF_SetRecordLengthProperly.vi"("Num Samples"=w1151, "VISA resource name"=refnum<visa-resource-name> "HV_Test_Scope") -> ()  [unwired: 1 in, 2 out]
                          }
                          frame #1 {
                            n168 = local write "Download"(TRUE ("Downloading")) -> ()
                            n169 = local write "Single"(FALSE ("Single")) -> ()
                            n170 = call "Agilent_Save_Array.vi"("Agilent Download"=TRUE, "Agilent Array In"=w1160, "File Path"=path "C:/HVTest/Local_Cap_Log_Scope") -> ("Agilent Array Out"=w1158:T2[])  [unwired: 1 in, 1 out]
                            n171 = local write "Agilent Array"(w1158) -> ()
                          }
                        }
                      }
                    }
                  }
                }
              }
            }
          }
        }
      }
      frame Disabled {
      }
    }
    n172 = To Word Integer(number="Max Number of Shots (Test intervals)") -> (16bit integer=w442:i16)
    n173 = To Variant(anything=w442) -> (Variant=w441:variant)
    n174 = case shown="0, Default" "HVPS Model" {
      tunnel: ["802L TDK PSU Voltage Rating (abs(Volts))" 12000 50000] -> w734
      tunnel: ["802L TDL PSU Peak Power (J/s)" 9000 9000] -> w757
      frame 2 {
      }
      frame 0, Default {
      }
      frame 1 {
      }
    }
    n175 = call-poly <userlib>:"Write TypeResolved.vi"("Handle"=w438, "SymbolName"=w439, "WData"=w441, "error constant"=w437) -> ("Write Status?"=w433:bool, "Has Matched?"=w434:bool, "error out"=w436:errorcluster)  [unwired: 8 in, 1 out]
    n176 = To Single Precision Float(number="Manual Charge Time (seconds)") -> (single precision float=w450:sgl)
    n177 = To Variant(anything=w450) -> (Variant=w449:variant)
    n178 = flat-sequence {
      tunnel: w790 -> [w1258]
      tunnel: w788 -> [w1259]
      tunnel: w789 -> [w1260]
      tunnel: [w1260] -> w800
      tunnel: [w1259] -> w799
      tunnel: [w1258] -> w798
      tunnel: [w1257] -> w797
      tunnel: w757 -> [w1256]
      tunnel: [w1263] -> w463
      tunnel: [w1266] -> w786
      tunnel: [w1265] -> w787
      tunnel: [w1264] -> w465
      tunnel: w800 -> [w1269]
      tunnel: w799 -> [w1268]
      tunnel: w798 -> [w1267]
      tunnel: w797 -> [w1262]
      tunnel: [w1261] -> w683
      frame #0 {
        # "Write Data"
        n179 = To Long Integer(number=w1256) -> (32bit integer=w1255:i32)
        n180 = To Variant(anything=w1255) -> (Variant=w1257:variant)
      }
      frame #1 {
        # "Resolve To TC"
        n181 = call <userlib>:"Resolve To TC Type.vi"("Handle"=w1267, "TypHdl"=w1268, "WData"=w1262, "error in"=w1269) -> ("Handle"=w1265:u32, "TypHdl"=w1266:u32, "bHasMatched"=w1261:bool, "ADSWData"=w1264:variant, "error out"=w1263:errorcluster)  [unwired: 7 in]
      }
    }
    n182 = flat-sequence {
      tunnel: w869 -> [w1408]
      tunnel: w868 -> [w1409]
      tunnel: w867 -> [w1410]
      tunnel: [w1410] -> w1015
      tunnel: [w1409] -> w1014
      tunnel: [w1408] -> w1013
      tunnel: [w1407] -> w1012
      tunnel: [w1413] -> w630
      tunnel: [w1416] -> w863
      tunnel: [w1415] -> w864
      tunnel: [w1414] -> w804
      tunnel: w1015 -> [w1419]
      tunnel: w1014 -> [w1418]
      tunnel: w1013 -> [w1417]
      tunnel: w1012 -> [w1412]
      tunnel: [w1411] -> w674
      frame #0 {
        # "Write Data"
        n183 = To Single Precision Float(number="Capacitance (uF)") -> (single precision float=w1406:sgl)
        n184 = To Variant(anything=w1406) -> (Variant=w1407:variant)
      }
      frame #1 {
        # "Resolve To TC"
        n185 = call <userlib>:"Resolve To TC Type.vi"("Handle"=w1417, "TypHdl"=w1418, "WData"=w1412, "error in"=w1419) -> ("Handle"=w1415:u32, "TypHdl"=w1416:u32, "bHasMatched"=w1411:bool, "ADSWData"=w1414:variant, "error out"=w1413:errorcluster)  [unwired: 7 in]
      }
    }
    n186 = flat-sequence {
      tunnel: w845 -> [w1378]
      tunnel: w844 -> [w1379]
      tunnel: w843 -> [w1380]
      tunnel: [w1380] -> w1007
      tunnel: [w1379] -> w1006
      tunnel: [w1378] -> w1005
      tunnel: [w1377] -> w1004
      tunnel: w734 -> [w1375]
      tunnel: [w1383] -> w624
      tunnel: [w1386] -> w839
      tunnel: [w1385] -> w840
      tunnel: [w1384] -> w802
      tunnel: w1007 -> [w1389]
      tunnel: w1006 -> [w1388]
      tunnel: w1005 -> [w1387]
      tunnel: w1004 -> [w1382]
      tunnel: [w1381] -> w678
      frame #0 {
        # "Write Data"
        n187 = To Long Integer(number=w1375) -> (32bit integer=w1376:i32)
        n188 = To Variant(anything=w1376) -> (Variant=w1377:variant)
      }
      frame #1 {
        # "Resolve To TC"
        n189 = call <userlib>:"Resolve To TC Type.vi"("Handle"=w1387, "TypHdl"=w1388, "WData"=w1382, "error in"=w1389) -> ("Handle"=w1385:u32, "TypHdl"=w1386:u32, "bHasMatched"=w1381:bool, "ADSWData"=w1384:variant, "error out"=w1383:errorcluster)  [unwired: 7 in]
      }
    }
    n190 = flat-sequence {
      tunnel: w877 -> [w1424]
      tunnel: [w1422] -> _
      tunnel: w875 -> [w1425]
      tunnel: [w1425] -> w1019
      tunnel: [w1422] -> w1018
      tunnel: [w1424] -> w1017
      tunnel: [w1423] -> w1016
      tunnel: w876 -> [w1422]
      tunnel: [w1428] -> w633
      tunnel: [w1431] -> w879
      tunnel: [w1430] -> w878
      tunnel: [w1429] -> w805
      tunnel: w1019 -> [w1434]
      tunnel: w1018 -> [w1433]
      tunnel: w1017 -> [w1432]
      tunnel: w1016 -> [w1427]
      tunnel: [w1426] -> w672
      frame #0 {
        # "Write Data"
        n191 = To Long Integer(number="Cycle Time (Sec)") -> (32bit integer=w1421:i32)
        n192 = To Variant(anything=w1421) -> (Variant=w1423:variant)
      }
      frame #1 {
        # "Resolve To TC"
        n193 = call <userlib>:"Resolve To TC Type.vi"("Handle"=w1432, "TypHdl"=w1433, "WData"=w1427, "error in"=w1434) -> ("Handle"=w1430:u32, "TypHdl"=w1431:u32, "bHasMatched"=w1426:bool, "ADSWData"=w1429:variant, "error out"=w1428:errorcluster)  [unwired: 7 in]
      }
    }
    n194 = flat-sequence {
      tunnel: w857 -> [w1393]
      tunnel: w856 -> [w1394]
      tunnel: w855 -> [w1395]
      tunnel: [w1395] -> w1011
      tunnel: [w1394] -> w1010
      tunnel: [w1393] -> w1009
      tunnel: [w1392] -> w1008
      tunnel: [w1398] -> w627
      tunnel: [w1401] -> w851
      tunnel: [w1400] -> w852
      tunnel: [w1399] -> w803
      tunnel: w1011 -> [w1404]
      tunnel: w1010 -> [w1403]
      tunnel: w1009 -> [w1402]
      tunnel: w1008 -> [w1397]
      tunnel: [w1396] -> w676
      frame #0 {
        # "Write Data"
        n195 = To Long Integer(number="Target Charge Volt (V) - Min 1500V - TEMPORARY LIMIT 12kV") -> (32bit integer=w1391:i32)
        n196 = To Variant(anything=w1391) -> (Variant=w1392:variant)
      }
      frame #1 {
        # "Resolve To TC"
        n197 = call <userlib>:"Resolve To TC Type.vi"("Handle"=w1402, "TypHdl"=w1403, "WData"=w1397, "error in"=w1404) -> ("Handle"=w1400:u32, "TypHdl"=w1401:u32, "bHasMatched"=w1396:bool, "ADSWData"=w1399:variant, "error out"=w1398:errorcluster)  [unwired: 7 in]
      }
    }
    n198 = flat-sequence {
      tunnel: w833 -> [w1363]
      tunnel: w832 -> [w1364]
      tunnel: w831 -> [w1365]
      tunnel: [w1365] -> w1003
      tunnel: [w1364] -> w1002
      tunnel: [w1363] -> w1001
      tunnel: [w1362] -> w1000
      tunnel: [w1368] -> w621
      tunnel: [w1371] -> w827
      tunnel: [w1370] -> w828
      tunnel: [w1369] -> w801
      tunnel: w1003 -> [w1374]
      tunnel: w1002 -> [w1373]
      tunnel: w1001 -> [w1372]
      tunnel: w1000 -> [w1367]
      tunnel: [w1366] -> w680
      frame #0 {
        # "Write Data"
        n199 = To Single Precision Float(number="Hold Time Before Shot (seconds)") -> (single precision float=w1361:sgl)
        n200 = To Variant(anything=w1361) -> (Variant=w1362:variant)
      }
      frame #1 {
        # "Resolve To TC"
        n201 = call <userlib>:"Resolve To TC Type.vi"("Handle"=w1372, "TypHdl"=w1373, "WData"=w1367, "error in"=w1374) -> ("Handle"=w1370:u32, "TypHdl"=w1371:u32, "bHasMatched"=w1366:bool, "ADSWData"=w1369:variant, "error out"=w1368:errorcluster)  [unwired: 7 in]
      }
    }
    n202 = To Word Integer(number="Cap 1 Fault Temp (Cel)") -> (16bit integer=w458:i16)
    n203 = flat-sequence {
      tunnel: w893 -> [w1273]
      tunnel: w892 -> [w1274]
      tunnel: w891 -> [w1275]
      tunnel: [w1275] -> w979
      tunnel: [w1274] -> w978
      tunnel: [w1273] -> w977
      tunnel: [w1272] -> w976
      tunnel: [w1278] -> w635
      tunnel: [w1281] -> w887
      tunnel: [w1280] -> w888
      tunnel: [w1279] -> w806
      tunnel: w979 -> [w1284]
      tunnel: w978 -> [w1283]
      tunnel: w977 -> [w1282]
      tunnel: w976 -> [w1277]
      tunnel: [w1276] -> w671
      frame #0 {
        # "Write Data"
        n204 = And(x="CLEAR FAULT", y="CLEAR FAULT") -> (x .and. y?=w1271:bool)
        n205 = To Variant(anything=w1271) -> (Variant=w1272:variant)
      }
      frame #1 {
        # "Resolve To TC"
        n206 = call <userlib>:"Resolve To TC Type.vi"("Handle"=w1282, "TypHdl"=w1283, "WData"=w1277, "error in"=w1284) -> ("Handle"=w1280:u32, "TypHdl"=w1281:u32, "bHasMatched"=w1276:bool, "ADSWData"=w1279:variant, "error out"=w1278:errorcluster)  [unwired: 7 in]
      }
    }
    n207 = flat-sequence {
      tunnel: w941 -> [w1333]
      tunnel: w940 -> [w1334]
      tunnel: w939 -> [w1335]
      tunnel: [w1335] -> w995
      tunnel: [w1334] -> w994
      tunnel: [w1333] -> w993
      tunnel: [w1332] -> w992
      tunnel: [w1338] -> w647
      tunnel: [w1341] -> w935
      tunnel: [w1340] -> w936
      tunnel: [w1339] -> w810
      tunnel: w995 -> [w1344]
      tunnel: w994 -> [w1343]
      tunnel: w993 -> [w1342]
      tunnel: w992 -> [w1337]
      tunnel: [w1336] -> w663
      frame #0 {
        # "Write Data"
        n208 = And(x="Hold", y="Hold") -> (x .and. y?=w1331:bool)
        n209 = To Variant(anything=w1331) -> (Variant=w1332:variant)
      }
      frame #1 {
        # "Resolve To TC"
        n210 = call <userlib>:"Resolve To TC Type.vi"("Handle"=w1342, "TypHdl"=w1343, "WData"=w1337, "error in"=w1344) -> ("Handle"=w1340:u32, "TypHdl"=w1341:u32, "bHasMatched"=w1336:bool, "ADSWData"=w1339:variant, "error out"=w1338:errorcluster)  [unwired: 7 in]
      }
    }
    n211 = flat-sequence {
      tunnel: w917 -> [w1303]
      tunnel: w916 -> [w1304]
      tunnel: w915 -> [w1305]
      tunnel: [w1305] -> w987
      tunnel: [w1304] -> w986
      tunnel: [w1303] -> w985
      tunnel: [w1302] -> w984
      tunnel: [w1308] -> w641
      tunnel: [w1311] -> w911
      tunnel: [w1310] -> w912
      tunnel: [w1309] -> w808
      tunnel: w987 -> [w1314]
      tunnel: w986 -> [w1313]
      tunnel: w985 -> [w1312]
      tunnel: w984 -> [w1307]
      tunnel: [w1306] -> w667
      frame #0 {
        # "Write Data"
        n212 = And(x="Shot", y="Shot") -> (x .and. y?=w1301:bool)
        n213 = To Variant(anything=w1301) -> (Variant=w1302:variant)
      }
      frame #1 {
        # "Resolve To TC"
        n214 = call <userlib>:"Resolve To TC Type.vi"("Handle"=w1312, "TypHdl"=w1313, "WData"=w1307, "error in"=w1314) -> ("Handle"=w1310:u32, "TypHdl"=w1311:u32, "bHasMatched"=w1306:bool, "ADSWData"=w1309:variant, "error out"=w1308:errorcluster)  [unwired: 7 in]
      }
    }
    n215 = flat-sequence {
      tunnel: w949 -> [w1349]
      tunnel: [w1345] -> _
      tunnel: w947 -> [w1350]
      tunnel: [w1350] -> w999
      tunnel: [w1345] -> w998
      tunnel: [w1349] -> w997
      tunnel: [w1348] -> w996
      tunnel: w948 -> [w1345]
      tunnel: [w1353] -> w650
      tunnel: [w1356] -> w951
      tunnel: [w1355] -> w950
      tunnel: [w1354] -> w811
      tunnel: w999 -> [w1359]
      tunnel: w998 -> [w1358]
      tunnel: w997 -> [w1357]
      tunnel: w996 -> [w1352]
      tunnel: [w1351] -> w661
      frame #0 {
        # "Write Data"
        n216 = And(x="Manual/Auto", y="Manual/Auto") -> (x .and. y?=w1347:bool)
        n217 = To Variant(anything=w1347) -> (Variant=w1348:variant)
      }
      frame #1 {
        # "Resolve To TC"
        n218 = call <userlib>:"Resolve To TC Type.vi"("Handle"=w1357, "TypHdl"=w1358, "WData"=w1352, "error in"=w1359) -> ("Handle"=w1355:u32, "TypHdl"=w1356:u32, "bHasMatched"=w1351:bool, "ADSWData"=w1354:variant, "error out"=w1353:errorcluster)  [unwired: 7 in]
      }
    }
    n219 = flat-sequence {
      tunnel: w929 -> [w1318]
      tunnel: w928 -> [w1319]
      tunnel: w927 -> [w1320]
      tunnel: [w1320] -> w991
      tunnel: [w1319] -> w990
      tunnel: [w1318] -> w989
      tunnel: [w1317] -> w988
      tunnel: [w1323] -> w644
      tunnel: [w1326] -> w923
      tunnel: [w1325] -> w924
      tunnel: [w1324] -> w809
      tunnel: w991 -> [w1329]
      tunnel: w990 -> [w1328]
      tunnel: w989 -> [w1327]
      tunnel: w988 -> [w1322]
      tunnel: [w1321] -> w665
      frame #0 {
        # "Write Data"
        n220 = And(x="Charge", y="Charge") -> (x .and. y?=w1316:bool)
        n221 = To Variant(anything=w1316) -> (Variant=w1317:variant)
      }
      frame #1 {
        # "Resolve To TC"
        n222 = call <userlib>:"Resolve To TC Type.vi"("Handle"=w1327, "TypHdl"=w1328, "WData"=w1322, "error in"=w1329) -> ("Handle"=w1325:u32, "TypHdl"=w1326:u32, "bHasMatched"=w1321:bool, "ADSWData"=w1324:variant, "error out"=w1323:errorcluster)  [unwired: 7 in]
      }
    }
    n223 = flat-sequence {
      tunnel: w905 -> [w1288]
      tunnel: w904 -> [w1289]
      tunnel: w903 -> [w1290]
      tunnel: [w1290] -> w983
      tunnel: [w1289] -> w982
      tunnel: [w1288] -> w981
      tunnel: [w1287] -> w980
      tunnel: [w1293] -> w638
      tunnel: [w1296] -> w899
      tunnel: [w1295] -> w900
      tunnel: [w1294] -> w807
      tunnel: w983 -> [w1299]
      tunnel: w982 -> [w1298]
      tunnel: w981 -> [w1297]
      tunnel: w980 -> [w1292]
      tunnel: [w1291] -> w669
      frame #0 {
        # "Write Data"
        n224 = And(x="HV Switch Mode", y="HV Switch Mode") -> (x .and. y?=w1286:bool)
        n225 = To Variant(anything=w1286) -> (Variant=w1287:variant)
      }
      frame #1 {
        # "Resolve To TC"
        n226 = call <userlib>:"Resolve To TC Type.vi"("Handle"=w1297, "TypHdl"=w1298, "WData"=w1292, "error in"=w1299) -> ("Handle"=w1295:u32, "TypHdl"=w1296:u32, "bHasMatched"=w1291:bool, "ADSWData"=w1294:variant, "error out"=w1293:errorcluster)  [unwired: 7 in]
      }
    }
    n227 = flat-sequence {
      tunnel: w965 -> [w1234]
      tunnel: w964 -> [w1235]
      tunnel: w963 -> [w1236]
      tunnel: [w1236] -> w725
      tunnel: [w1235] -> w724
      tunnel: [w1234] -> w723
      tunnel: [w1233] -> w722
      tunnel: w725 -> [w1245]
      tunnel: w724 -> [w1244]
      tunnel: w723 -> [w1243]
      tunnel: w722 -> [w1238]
      tunnel: [w1239] -> w653
      tunnel: [w1242] -> w959
      tunnel: [w1241] -> w960
      tunnel: [w1240] -> w721
      tunnel: [w1237] -> w659
      frame #0 {
        # "Write Data"
        n228 = And(x="STOP", y="STOP") -> (x .and. y?=w1232:bool)
        n229 = To Variant(anything=w1232) -> (Variant=w1233:variant)
      }
      frame #1 {
        # "Resolve To TC"
        n230 = call <userlib>:"Resolve To TC Type.vi"("Handle"=w1243, "TypHdl"=w1244, "WData"=w1238, "error in"=w1245) -> ("Handle"=w1241:u32, "TypHdl"=w1242:u32, "bHasMatched"=w1237:bool, "ADSWData"=w1240:variant, "error out"=w1239:errorcluster)  [unwired: 7 in]
      }
    }
    n231 = flat-sequence {
      tunnel: w609 -> [w1181]
      tunnel: w608 -> [w1177]
      tunnel: w607 -> [w1182]
      tunnel: [w1182] -> w618
      tunnel: [w1177] -> w617
      tunnel: [w1181] -> w616
      tunnel: [w1180] -> w615
      tunnel: [w1185] -> w460
      tunnel: [w1188] -> w602
      tunnel: [w1187] -> w603
      tunnel: [w1186] -> w606
      tunnel: w618 -> [w1191]
      tunnel: w617 -> [w1190]
      tunnel: w616 -> [w1189]
      tunnel: w615 -> [w1184]
      tunnel: [w1183] -> w600
      frame #0 {
        # "Write Data"
        n232 = And(x="Reset Test Number", y="Reset Test Number") -> (x .and. y?=w1179:bool)
        n233 = To Variant(anything=w1179) -> (Variant=w1180:variant)
      }
      frame #1 {
        # "Resolve To TC"
        n234 = call <userlib>:"Resolve To TC Type.vi"("Handle"=w1189, "TypHdl"=w1190, "WData"=w1184, "error in"=w1191) -> ("Handle"=w1187:u32, "TypHdl"=w1188:u32, "bHasMatched"=w1183:bool, "ADSWData"=w1186:variant, "error out"=w1185:errorcluster)  [unwired: 7 in]
      }
    }
    n235 = flat-sequence {
      tunnel: w975 -> [w1200]
      tunnel: w974 -> [w1201]
      tunnel: w971 -> [w1202]
      tunnel: [w1202] -> w720
      tunnel: [w1201] -> w719
      tunnel: [w1200] -> w718
      tunnel: [w1199] -> w717
      tunnel: [w1197] -> _
      tunnel: [w1197] -> w716
      tunnel: w733 -> [w1197]
      tunnel: w732 -> [w1196]
      tunnel: [w1196] -> w715
      tunnel: w731 -> [w1195]
      tunnel: [w1195] -> w714
      tunnel: w730 -> [w1194]
      tunnel: [w1194] -> w713
      tunnel: w729 -> [w1193]
      tunnel: [w1193] -> w712
      tunnel: ["START"] -> w543
      tunnel: w720 -> [w1216]
      tunnel: w719 -> [w1215]
      tunnel: w718 -> [w1214]
      tunnel: w717 -> [w1209]
      tunnel: [w1210] -> w711
      tunnel: [w1213] -> w710
      tunnel: [w1212] -> w709
      tunnel: [w1211] -> w708
      tunnel: [w1208] -> w707
      tunnel: w716 -> [w1207]
      tunnel: [w1207] -> w706
      tunnel: w715 -> [w1206]
      tunnel: [w1206] -> w705
      tunnel: w714 -> [w1205]
      tunnel: [w1205] -> w704
      tunnel: w713 -> [w1204]
      tunnel: [w1204] -> w703
      tunnel: [w1203] -> w702
      tunnel: w712 -> [w1203]
      tunnel: [w1227] -> w685
      tunnel: [w1228] -> w973
      tunnel: [w1229] -> w972
      tunnel: [w1230] -> w656
      tunnel: w711 -> [w1230]
      tunnel: w710 -> [w1229]
      tunnel: w709 -> [w1228]
      tunnel: w708 -> [w1219]
      tunnel: w707 -> [w1227]
      tunnel: w706 -> [w1226]
      tunnel: w705 -> [w1225]
      tunnel: w704 -> [w1224]
      tunnel: w703 -> [w1223]
      tunnel: w702 -> [w1222]
      tunnel: [w1221] -> w728
      tunnel: [w1220] -> w727
      tunnel: [w1218] -> w657
      tunnel: [w1217] -> w700
      frame #0 {
        # "Write Data"
        n236 = And(x="START", y="START") -> (x .and. y?=w1198:bool)
        n237 = To Variant(anything=w1198) -> (Variant=w1199:variant)
      }
      frame #1 {
        # "Resolve To TC"
        n238 = call <userlib>:"Resolve To TC Type.vi"("Handle"=w1214, "TypHdl"=w1215, "WData"=w1209, "error in"=w1216) -> ("Handle"=w1212:u32, "TypHdl"=w1213:u32, "bHasMatched"=w1208:bool, "ADSWData"=w1211:variant, "error out"=w1210:errorcluster)  [unwired: 7 in]
      }
      frame #2 {
        # "Write"
        n239 = call <userlib>:"Send Writer-Request.vi"("Handle"=w1226, "SymbolName"=w1225, "WriterMode"=w1224, "WriteHandle"=w1223, "error constant"=w1222, "ADS Write Data"=w1219) -> ("Handle"=w1221:u32, "WriteHandle"=w1220:u32, "Write status?"=w1217:bool, "error IO"=w1218:errorcluster)  [unwired: 5 in, 1 out]
      }
    }
    n240 = To Variant(anything=w458) -> (Variant=w457:variant)
    n241 = call-poly <userlib>:"Write TypeResolved.vi"("Handle"=w438, "SymbolName"=w448, "WData"=w449, "error constant"=w447) -> ("Write Status?"=w443:bool, "Has Matched?"=w444:bool, "error out"=w446:errorcluster)  [unwired: 8 in, 1 out]
    n242 = call-poly <userlib>:"Write TypeResolved.vi"("Handle"=w438, "SymbolName"=w455, "WData"=w457, "error constant"=w456) -> ("Write Status?"=w452:bool, "Has Matched?"=w454:bool, "error out"=w453:errorcluster)  [unwired: 8 in, 1 out]
    n243 = To Single Precision Float(number="Duty Cycle") -> (single precision float=w502:sgl)
    n244 = And(x="Voltage Held by PSU", y="Voltage Held by PSU") -> (x .and. y?=w490:bool)
    n245 = And(x="Current Control", y="Current Control") -> (x .and. y?=w509:bool)
    n246 = To Variant(anything=w502) -> (Variant=w506:variant)
    n247 = And(x="Dump", y="Dump") -> (x .and. y?=w518:bool)
    n248 = To Variant(anything=w490) -> (Variant=w488:variant)
    n249 = To Variant(anything=w509) -> (Variant=w507:variant)
    n250 = To Variant(anything=w518) -> (Variant=w519:variant)
    n251 = call-poly <userlib>:"Write TypeResolved.vi"("Handle"=w438, "SymbolName"=w491, "WData"=w488, "error constant"=w487) -> ("Write Status?"=w480:bool, "Has Matched?"=w481:bool, "error out"=w486:errorcluster)  [unwired: 8 in, 1 out]
    n252 = flat-sequence {
      tunnel: w826 -> [w1566]
      tunnel: w825 -> [w1564]
      tunnel: w824 -> [w1562]
      tunnel: [w1565] -> w1054
      tunnel: [w1563] -> w1053
      tunnel: [w1561] -> w1052
      tunnel: [w1560] -> w1051
      tunnel: [w1559] -> w1050
      tunnel: [w1558] -> w1049
      tunnel: [w1557] -> w1048
      tunnel: [w1556] -> w1047
      tunnel: [w1555] -> w1046
      tunnel: [w1554] -> w1045
      tunnel: [w1553] -> w1044
      tunnel: w822 -> [w1552]
      tunnel: w821 -> [w1551]
      tunnel: w820 -> [w1550]
      tunnel: w819 -> [w1549]
      tunnel: w818 -> [w1548]
      tunnel: w817 -> [w1547]
      tunnel: [w1546] -> w1043
      tunnel: [w1545] -> w1042
      tunnel: [w1544] -> w1041
      tunnel: [w1543] -> w1040
      tunnel: [w1542] -> w1039
      tunnel: [w1541] -> w1038
      tunnel: [w1540] -> w1037
      tunnel: [w1539] -> w1036
      tunnel: [w1538] -> w1035
      tunnel: [w1537] -> w1034
      tunnel: [w1536] -> w1033
      tunnel: [w1535] -> w1032
      tunnel: [w1534] -> w1031
      tunnel: [w1533] -> w1030
      tunnel: [w1532] -> w1029
      tunnel: [w1531] -> w1028
      tunnel: [w1530] -> w1027
      tunnel: [w1529] -> w1026
      tunnel: [w1528] -> w1025
      tunnel: [w1527] -> w1024
      tunnel: [w1526] -> w1023
      tunnel: [w1525] -> w1022
      tunnel: [w1524] -> w1021
      tunnel: [w1523] -> w1020
      tunnel: w784 -> [w1522]
      tunnel: [w1521] -> w783
      tunnel: [w1520] -> w782
      tunnel: [w1519] -> w781
      tunnel: [w1518] -> w780
      tunnel: [w1517] -> w779
      tunnel: w777 -> [w1436]
      tunnel: [w1516] -> w776
      tunnel: w774 -> [w1515]
      tunnel: [w1514] -> w773
      tunnel: [w1513] -> w772
      tunnel: [w1512] -> w771
      tunnel: w770 -> [w1511]
      tunnel: w769 -> [w1510]
      tunnel: [w1509] -> w768
      tunnel: [w1508] -> w767
      tunnel: [w1507] -> w766
      tunnel: [w1506] -> w765
      tunnel: [w1505] -> w764
      tunnel: [w1504] -> w763
      tunnel: [w1503] -> w762
      tunnel: [w1502] -> w761
      tunnel: w753 -> [w1501]
      tunnel: w752 -> [w1500]
      tunnel: w751 -> [w1499]
      tunnel: [w1498] -> w750
      tunnel: [w1497] -> w749
      tunnel: [w1496] -> w748
      tunnel: [w1495] -> w747
      tunnel: [w1494] -> w746
      tunnel: [w1493] -> w745
      tunnel: [w1492] -> w744
      tunnel: [w1491] -> w743
      tunnel: [w1490] -> w742
      tunnel: [w1489] -> w741
      tunnel: [w1488] -> w740
      tunnel: [w1487] -> w739
      tunnel: [w1440] -> _
      tunnel: w726 -> [w1440]
      tunnel: [w1486] -> w594
      tunnel: [w1485] -> w593
      tunnel: [w1484] -> w592
      tunnel: w591 -> [w1483]
      tunnel: [w1482] -> w587
      tunnel: w586 -> [w1481]
      tunnel: [w1480] -> w585
      tunnel: [w1479] -> w584
      tunnel: [w1478] -> w583
      tunnel: [w1477] -> w582
      tunnel: w581 -> [w1476]
      tunnel: w580 -> [w1475]
      tunnel: w579 -> [w1474]
      tunnel: [w1473] -> w578
      tunnel: [w1472] -> w577
      tunnel: [w1471] -> w575
      tunnel: [w1470] -> w573
      tunnel: [w1469] -> w572
      tunnel: [w1468] -> w571
      tunnel: [w1467] -> w570
      tunnel: [w1466] -> w567
      tunnel: w566 -> [w1465]
      tunnel: [w1464] -> w565
      tunnel: [w1463] -> w564
      tunnel: [w1462] -> w563
      tunnel: w541 -> [w1461]
      tunnel: w540 -> [w1460]
      tunnel: [w1459] -> w539
      tunnel: [w1458] -> w538
      tunnel: [w1457] -> w537
      tunnel: [w1456] -> w536
      tunnel: [w1455] -> w535
      tunnel: [w1454] -> w534
      tunnel: w533 -> [w1453]
      tunnel: [w1452] -> w532
      tunnel: [w1451] -> w531
      tunnel: [w1450] -> w530
      tunnel: w516 -> [w1449]
      tunnel: [w1448] -> w515
      tunnel: [w1447] -> w514
      tunnel: [w1446] -> w513
      tunnel: [w1445] -> w475
      tunnel: [w1444] -> w474
      tunnel: w473 -> [w1443]
      tunnel: w472 -> [w1441]
      tunnel: [w1442] -> w471
      tunnel: [w1439] -> w470
      tunnel: [w1438] -> w469
      tunnel: [w1437] -> w468
      tunnel: [w1435] -> w462
      tunnel: w1054 -> [w1779]
      tunnel: w1053 -> [w1792]
      tunnel: w1052 -> [_]
      tunnel: w1051 -> [w1778]
      tunnel: w1050 -> [w1777]
      tunnel: w1049 -> [w1607]
      tunnel: [w1707] -> w823
      tunnel: w1048 -> [w1791]
      tunnel: w1047 -> [w1793]
      tunnel: w1046 -> [w1795]
      tunnel: w1045 -> [w1616]
      tunnel: w1044 -> [_]
      tunnel: w1043 -> [w1774]
      tunnel: w1042 -> [w1789]
      tunnel: w1041 -> [w1787]
      tunnel: w1040 -> [w1785]
      tunnel: w1039 -> [w1783]
      tunnel: w1038 -> [w1781]
      tunnel: [w1720] -> w816
      tunnel: w1037 -> [w1773]
      tunnel: w1036 -> [w1772]
      tunnel: w1035 -> [w1771]
      tunnel: w1034 -> [w1770]
      tunnel: w1033 -> [w1769]
      tunnel: w1032 -> [w1768]
      tunnel: w1031 -> [_]
      tunnel: w1030 -> [w1605]
      tunnel: w1029 -> [_]
      tunnel: w1028 -> [w1603]
      tunnel: w1027 -> [_]
      tunnel: w1026 -> [w1601]
      tunnel: w1025 -> [_]
      tunnel: w1024 -> [w1599]
      tunnel: w1023 -> [_]
      tunnel: w1022 -> [w1597]
      tunnel: w1021 -> [_]
      tunnel: w1020 -> [w1595]
      tunnel: [w1722] -> w815
      tunnel: [w1724] -> w814
      tunnel: [w1726] -> w813
      tunnel: [w1728] -> w812
      tunnel: w783 -> [w1593]
      tunnel: w782 -> [w1759]
      tunnel: w781 -> [_]
      tunnel: w780 -> [w1691]
      tunnel: w779 -> [w1755]
      tunnel: [w1711] -> w778
      tunnel: w776 -> [w1758]
      tunnel: [w1709] -> w775
      tunnel: w773 -> [w1757]
      tunnel: w772 -> [w1569]
      tunnel: w771 -> [_]
      tunnel: w768 -> [w1753]
      tunnel: w767 -> [w1752]
      tunnel: w766 -> [w1749]
      tunnel: w765 -> [w1748]
      tunnel: w764 -> [w1747]
      tunnel: w763 -> [w1746]
      tunnel: w762 -> [_]
      tunnel: w761 -> [_]
      tunnel: [w1713] -> w760
      tunnel: [w1715] -> w759
      tunnel: [w1730] -> w756
      tunnel: [w1733] -> w755
      tunnel: [w1732] -> w754
      tunnel: w750 -> [w1744]
      tunnel: w749 -> [w1742]
      tunnel: w748 -> [w1740]
      tunnel: w747 -> [w1611]
      tunnel: w746 -> [w1609]
      tunnel: w745 -> [w1613]
      tunnel: w744 -> [w1739]
      tunnel: w743 -> [w1738]
      tunnel: w742 -> [w1737]
      tunnel: w741 -> [_]
      tunnel: w740 -> [_]
      tunnel: w739 -> [_]
      tunnel: [w1718] -> w738
      tunnel: [w1716] -> w737
      tunnel: [w1705] -> w736
      tunnel: [w1706] -> w432
      tunnel: [w1697] -> w619
      tunnel: [w1699] -> w595
      tunnel: w594 -> [w1615]
      tunnel: w593 -> [w1702]
      tunnel: w592 -> [_]
      tunnel: [w1700] -> w590
      tunnel: w587 -> [w1694]
      tunnel: w585 -> [w1689]
      tunnel: w584 -> [w1686]
      tunnel: w583 -> [w1684]
      tunnel: w582 -> [w1671]
      tunnel: w578 -> [w1591]
      tunnel: w577 -> [w1683]
      tunnel: [w1682] -> w576
      tunnel: w575 -> [w1681]
      tunnel: [w1680] -> w574
      tunnel: w573 -> [w1679]
      tunnel: w572 -> [w1587]
      tunnel: w571 -> [w1678]
      tunnel: w570 -> [w1585]
      tunnel: [w1677] -> w569
      tunnel: [w1676] -> w568
      tunnel: w567 -> [w1589]
      tunnel: [w1675] -> w550
      tunnel: [w1674] -> w548
      tunnel: [w1673] -> w558
      tunnel: w565 -> [w1667]
      tunnel: w564 -> [w1583]
      tunnel: w563 -> [w1669]
      tunnel: [w1668] -> w562
      tunnel: w539 -> [w1663]
      tunnel: w538 -> [w1581]
      tunnel: w537 -> [w1665]
      tunnel: w536 -> [w1664]
      tunnel: w535 -> [w1659]
      tunnel: w534 -> [w1579]
      tunnel: w532 -> [w1645]
      tunnel: w531 -> [w1577]
      tunnel: w530 -> [w1658]
      tunnel: [w1651] -> w529
      tunnel: [w1650] -> w528
      tunnel: [w1649] -> w527
      tunnel: [w1648] -> w526
      tunnel: w515 -> [w1626]
      tunnel: w514 -> [w1643]
      tunnel: w513 -> [w1575]
      tunnel: [w1642] -> w512
      tunnel: w475 -> [w1573]
      tunnel: w474 -> [w1627]
      tunnel: w471 -> [w1622]
      tunnel: w470 -> [w1624]
      tunnel: w469 -> [w1623]
      tunnel: w468 -> [w1571]
      tunnel: [w1618] -> w467
      tunnel: [w1617] -> w466
      tunnel: w462 -> [_]
      frame #0 {
        # "Read and Resolve Data."
        # "Read/Resolve Symbol N"
        # "Read Data and Resolve Type"
        n253 = call-poly <userlib>:"Read TypeResolved.vi"("Handle"=w1440, "SymbolName"=w1510, "error constant"=w1436) -> ("Handle"=w1503:u32, "Read Status?"=w1508:bool, "RData"=w1504:variant, "error out"=w1507:errorcluster)  [unwired: 9 in]
        n254 = call-poly <userlib>:"Read TypeResolved.vi"("Handle"=w1440, "SymbolName"=w1511, "error constant"=w1436) -> ("Handle"=w1502:u32, "Read Status?"=w1509:bool, "RData"=w1505:variant, "error out"=w1506:errorcluster)  [unwired: 9 in]
        n255 = call-poly <userlib>:"Read TypeResolved.vi"("Handle"=w1440, "SymbolName"=w1564, "error constant"=w1436) -> ("Handle"=w1554:u32, "Read Status?"=w1556:bool, "RData"=w1560:variant, "error out"=w1565:errorcluster)  [unwired: 9 in]
        n256 = call-poly <userlib>:"Read TypeResolved.vi"("Handle"=w1440, "SymbolName"=w1515, "error constant"=w1436) -> ("Handle"=w1512:u32, "Read Status?"=w1514:bool, "RData"=w1513:variant, "error out"=w1517:errorcluster)  [unwired: 9 in]
        n257 = call-poly <userlib>:"Read TypeResolved.vi"("Handle"=w1440, "SymbolName"=w1566, "error constant"=w1436) -> ("Handle"=w1553:u32, "Read Status?"=w1555:bool, "RData"=w1559:variant, "error out"=w1516:errorcluster)  [unwired: 9 in]
        n258 = call-poly <userlib>:"Read TypeResolved.vi"("Handle"=w1440, "SymbolName"=w1443, "error constant"=w1436) -> ("Read Status?"=w1442:bool, "RData"=w1445:variant, "error out"=w1444:errorcluster)  [unwired: 9 in, 1 out]
        n259 = call-poly <userlib>:"Read TypeResolved.vi"("Handle"=w1440, "SymbolName"=w1562, "error constant"=w1436) -> ("Handle"=w1561:u32, "Read Status?"=w1557:bool, "RData"=w1558:variant, "error out"=w1563:errorcluster)  [unwired: 9 in]
        n260 = call-poly <userlib>:"Read TypeResolved.vi"("Handle"=w1440, "SymbolName"=w1552, "error constant"=w1436) -> ("Handle"=w1534:u32, "Read Status?"=w1541:bool, "RData"=w1533:variant, "error out"=w1540:errorcluster)  [unwired: 9 in]
        n261 = call-poly <userlib>:"Read TypeResolved.vi"("Handle"=w1440, "SymbolName"=w1453, "error constant"=w1436) -> ("Read Status?"=w1452:bool, "RData"=w1451:variant, "error out"=w1450:errorcluster)  [unwired: 9 in, 1 out]
        n262 = call-poly <userlib>:"Read TypeResolved.vi"("Handle"=w1440, "SymbolName"=w1441, "error constant"=w1436) -> ("Read Status?"=w1438:bool, "RData"=w1437:variant, "error out"=w1439:errorcluster)  [unwired: 9 in, 1 out]
        n263 = call-poly <userlib>:"Read TypeResolved.vi"("Handle"=w1440, "SymbolName"=w1449, "error constant"=w1436) -> ("Read Status?"=w1448:bool, "RData"=w1446:variant, "error out"=w1447:errorcluster)  [unwired: 9 in, 1 out]
        n264 = call-poly <userlib>:"Read TypeResolved.vi"("Handle"=w1440, "SymbolName"=w1550, "error constant"=w1436) -> ("Handle"=w1530:u32, "Read Status?"=w1543:bool, "RData"=w1529:variant, "error out"=w1538:errorcluster)  [unwired: 9 in]
        n265 = call-poly <userlib>:"Read TypeResolved.vi"("Handle"=w1440, "SymbolName"=w1548, "error constant"=w1436) -> ("Handle"=w1526:u32, "Read Status?"=w1545:bool, "RData"=w1525:variant, "error out"=w1536:errorcluster)  [unwired: 9 in]
        n266 = call-poly <userlib>:"Read TypeResolved.vi"("Handle"=w1440, "SymbolName"=w1465, "error constant"=w1436) -> ("Read Status?"=w1464:bool, "RData"=w1463:variant, "error out"=w1462:errorcluster)  [unwired: 9 in, 1 out]
        n267 = call-poly <userlib>:"Read TypeResolved.vi"("Handle"=w1440, "SymbolName"=w1461, "error constant"=w1436) -> ("Read Status?"=w1459:bool, "RData"=w1458:variant, "error out"=w1457:errorcluster)  [unwired: 9 in, 1 out]
        n268 = call-poly <userlib>:"Read TypeResolved.vi"("Handle"=w1440, "SymbolName"=w1460, "error constant"=w1436) -> ("Read Status?"=w1455:bool, "RData"=w1454:variant, "error out"=w1456:errorcluster)  [unwired: 9 in, 1 out]
        n269 = call-poly <userlib>:"Read TypeResolved.vi"("Handle"=w1440, "SymbolName"=w1551, "error constant"=w1436) -> ("Handle"=w1532:u32, "Read Status?"=w1542:bool, "RData"=w1531:variant, "error out"=w1539:errorcluster)  [unwired: 9 in]
        n270 = call-poly <userlib>:"Read TypeResolved.vi"("Handle"=w1440, "SymbolName"=w1549, "error constant"=w1436) -> ("Handle"=w1528:u32, "Read Status?"=w1544:bool, "RData"=w1527:variant, "error out"=w1537:errorcluster)  [unwired: 9 in]
        n271 = call-poly <userlib>:"Read TypeResolved.vi"("Handle"=w1440, "SymbolName"=w1547, "error constant"=w1436) -> ("Handle"=w1524:u32, "Read Status?"=w1546:bool, "RData"=w1523:variant, "error out"=w1535:errorcluster)  [unwired: 9 in]
        n272 = call-poly <userlib>:"Read TypeResolved.vi"("Handle"=w1440, "SymbolName"=w1522, "error constant"=w1436) -> ("Handle"=w1519:u32, "Read Status?"=w1518:bool, "RData"=w1521:variant, "error out"=w1520:errorcluster)  [unwired: 9 in]
        n273 = call-poly <userlib>:"Read TypeResolved.vi"("Handle"=w1440, "SymbolName"=w1481, "error constant"=w1436) -> ("Handle"=w1435:u32, "Read Status?"=w1480:bool, "RData"=w1473:variant, "error out"=w1472:errorcluster)  [unwired: 9 in]
        n274 = call-poly <userlib>:"Read TypeResolved.vi"("Handle"=w1440, "SymbolName"=w1476, "error constant"=w1436) -> ("Read Status?"=w1479:bool, "RData"=w1466:variant, "error out"=w1471:errorcluster)  [unwired: 9 in, 1 out]
        n275 = call-poly <userlib>:"Read TypeResolved.vi"("Handle"=w1440, "SymbolName"=w1474, "error constant"=w1436) -> ("Read Status?"=w1477:bool, "RData"=w1467:variant, "error out"=w1468:errorcluster)  [unwired: 9 in, 1 out]
        n276 = call-poly <userlib>:"Read TypeResolved.vi"("Handle"=w1440, "SymbolName"=w1475, "error constant"=w1436) -> ("Read Status?"=w1478:bool, "RData"=w1469:variant, "error out"=w1470:errorcluster)  [unwired: 9 in, 1 out]
        n277 = call-poly <userlib>:"Read TypeResolved.vi"("Handle"=w1440, "SymbolName"=w1501, "error constant"=w1436) -> ("Handle"=w1489:u32, "Read Status?"=w1498:bool, "RData"=w1494:variant, "error out"=w1490:errorcluster)  [unwired: 9 in]
        n278 = call-poly <userlib>:"Read TypeResolved.vi"("Handle"=w1440, "SymbolName"=w1500, "error constant"=w1436) -> ("Handle"=w1488:u32, "Read Status?"=w1497:bool, "RData"=w1495:variant, "error out"=w1491:errorcluster)  [unwired: 9 in]
        n279 = call-poly <userlib>:"Read TypeResolved.vi"("Handle"=w1440, "SymbolName"=w1483, "error constant"=w1436) -> ("Handle"=w1484:u32, "Read Status?"=w1482:bool, "RData"=w1486:variant, "error out"=w1485:errorcluster)  [unwired: 9 in]
        n280 = call-poly <userlib>:"Read TypeResolved.vi"("Handle"=w1440, "SymbolName"=w1499, "error constant"=w1436) -> ("Handle"=w1487:u32, "Read Status?"=w1496:bool, "RData"=w1493:variant, "error out"=w1492:errorcluster)  [unwired: 9 in]
      }
      frame #1 {
        # "Cast Symbol N to LabVIEW Type"
        # "Variant To Data"
        n281 = To Variant(anything=w1571) -> (Variant=w1570:variant)
        n282 = To Variant(anything=w1613) -> (Variant=w1612:variant)
        n283 = To Variant(anything=w1585) -> (Variant=w1584:variant)
        n284 = To Variant(anything=w1611) -> (Variant=w1610:variant)
        n285 = To Variant(anything=w1579) -> (Variant=w1578:variant)
        n286 = To Variant(anything=w1581) -> (Variant=w1580:variant)
        n287 = To Variant(anything=w1573) -> (Variant=w1572:variant)
        n288 = To Variant(anything=w1583) -> (Variant=w1582:variant)
        n289 = To Variant(anything=w1575) -> (Variant=w1574:variant)
        n290 = To Variant(anything=w1577) -> (Variant=w1576:variant)
        n291 = To Variant(anything=w1609) -> (Variant=w1608:variant)
        n292 = To Variant(anything=w1593) -> (Variant=w1592:variant)
        n293 = To Variant(anything=w1591) -> (Variant=w1590:variant)
        n294 = To Variant(anything=w1589) -> (Variant=w1588:variant)
        n295 = To Variant(anything=w1603) -> (Variant=w1602:variant)
        n296 = To Variant(anything=w1569) -> (Variant=w1568:variant)
        n297 = To Variant(anything=w1587) -> (Variant=w1586:variant)
        n298 = To Variant(anything=w1607) -> (Variant=w1606:variant)
        n299 = To Variant(anything=w1605) -> (Variant=w1604:variant)
        n300 = To Variant(anything=w1595) -> (Variant=w1594:variant)
        n301 = To Variant(anything=w1615) -> (Variant=w1614:variant)
        n302 = To Variant(anything=w1601) -> (Variant=w1600:variant)
        n303 = To Variant(anything=w1597) -> (Variant=w1596:variant)
        n304 = To Variant(anything=w1599) -> (Variant=w1598:variant)
        n305 = And(x=w1622, y=w1623) -> (x .and. y?=w1621:bool)
        n306 = And(x=w1626, y=w1621) -> (x .and. y?=w1625:bool)
        n307 = Variant To Data(error in=w1627, Variant=w1572) -> (data=→"Test Interval (Sec)":i32, error out=w1618:errorcluster)  [unwired: 1 in]
        n308 = Variant To Data(error in=w1624, Variant=w1570) -> (data=→"Test Interval Fault":bool, error out=w1617:errorcluster)  [unwired: 1 in]
        n309 = And(x=w1645, y=w1625) -> (x .and. y?=w1644:bool)
        n310 = And(x=w1659, y=w1644) -> (x .and. y?=w1660:bool)
        n311 = And(x=w1663, y=w1660) -> (x .and. y?=w1662:bool)
        n312 = And(x=w1667, y=w1662) -> (x .and. y?=w1666:bool)
        n313 = And(x=w1671, y=w1666) -> (x .and. y?=w1670:bool)
        n314 = And(x=w1684, y=w1670) -> (x .and. y?=w1685:bool)
        n315 = And(x=w1686, y=w1685) -> (x .and. y?=w1687:bool)
        n316 = And(x=w1689, y=w1687) -> (x .and. y?=w1688:bool)
        n317 = And(x=w1691, y=w1688) -> (x .and. y?=w1690:bool)
        n318 = And(x=w1774, y=w1690) -> (x .and. y?=w1790:bool)
        n319 = And(x=w1789, y=w1790) -> (x .and. y?=w1788:bool)
        n320 = And(x=w1787, y=w1788) -> (x .and. y?=w1786:bool)
        n321 = And(x=w1785, y=w1786) -> (x .and. y?=w1784:bool)
        n322 = And(x=w1783, y=w1784) -> (x .and. y?=w1782:bool)
        n323 = And(x=w1781, y=w1782) -> (x .and. y?=w1780:bool)
        n324 = And(x=w1791, y=w1780) -> (x .and. y?=w1745:bool)
        n325 = And(x=w1744, y=w1745) -> (x .and. y?=w1743:bool)
        n326 = And(x=w1742, y=w1743) -> (x .and. y?=w1741:bool)
        n327 = And(x=w1740, y=w1741) -> (x .and. y?=w1693:bool)
        n328 = And(x=w1694, y=w1693) -> (x .and. y?=w1692:bool)
        n329 = And(x=w1752, y=w1692) -> (x .and. y?=w1751:bool)
        n330 = And(x=w1753, y=w1751) -> (x .and. y?=w1750:bool)
        n331 = And(x=w1757, y=w1750) -> (x .and. y?=w1756:bool)
        n332 = And(x=w1795, y=w1756) -> (x .and. y?=w1794:bool)
        n333 = Variant To Data(error in=w1702, Variant=w1614) -> (data=→"Cap 1 Voltage (HVPS)":i16, error out=w1700:errorcluster)  [unwired: 1 in]
        n334 = Variant To Data(error in=w1773, Variant=w1604) -> (data=→"Discharge Fault":bool, error out=w1722:errorcluster)  [unwired: 1 in]
        n335 = Variant To Data(error in=w1792, Variant=w1606) -> (data=→"Charge Fault":bool, error out=w1720:errorcluster)  [unwired: 1 in]
        n336 = Variant To Data(error in=w1771, Variant=w1600) -> (data=→"Cap 1 Temp\nExceeded Fault":bool, error out=w1726:errorcluster)  [unwired: 1 in]
        n337 = And(x=w1793, y=w1794) -> (x .and. y?=→"Read Status":bool)
        n338 = Variant To Data(error in=w1772, Variant=w1602) -> (data=→"Hold Fault":bool, error out=w1724:errorcluster)  [unwired: 1 in]
        n339 = Variant To Data(error in=w1739, Variant=w1612) -> (data=→"Load Temperature":i16, error out=w1705:errorcluster)  [unwired: 1 in]
        n340 = Variant To Data(error in=w1770, Variant=w1598) -> (data=→"Ambient Temp\nExceeded Fault":bool, error out=w1728:errorcluster)  [unwired: 1 in]
        n341 = Variant To Data(error in=w1769, Variant=w1596) -> (data=→"PSU Fault":bool, error out=w1730:errorcluster)  [unwired: 1 in]
        n342 = Variant To Data(error in=w1768, Variant=w1594) -> (data=→"Control Sys Fault":bool, error out=w1732:errorcluster)  [unwired: 1 in]
        n343 = Variant To Data(error in=w1759, Variant=w1592) -> (data=→"test Running":bool, error out=w1733:errorcluster)  [unwired: 1 in]
        n344 = Variant To Data(error in=w1737, Variant=w1608) -> (data=→"Ambient Temp":i16, error out=w1718:errorcluster)  [unwired: 1 in]
        n345 = Variant To Data(error in=w1678, Variant=w1584) -> (data=w1673:bool, error out=w1676:errorcluster)  [unwired: 1 in]
        "Soft Exception" <- w1673
        n346 = Variant To Data(error in=w1669, Variant=w1582) -> (data=w1567:bool, error out=w1651:errorcluster)  [unwired: 1 in]
        "EOC" <- w1567
        n347 = Variant To Data(error in=w1738, Variant=w1610) -> (data=→"Soft Dump Temp":i16, error out=w1716:errorcluster)  [unwired: 1 in]
        n348 = Variant To Data(error in=w1683, Variant=w1590) -> (data=w1668:bool, error out=w1682:errorcluster)  [unwired: 1 in]
        "Softdump FB Fault" <- w1668
        n349 = Variant To Data(error in=w1679, Variant=w1586) -> (data=w1674:bool, error out=w1677:errorcluster)  [unwired: 1 in]
        "PSU HV FB Fault" <- w1674
        n350 = Variant To Data(error in=w1665, Variant=w1580) -> (data=w1639:bool, error out=w1650:errorcluster)  [unwired: 1 in]
        "SCR Ready" <- w1639
        n351 = Variant To Data(error in=w1664, Variant=w1578) -> (data=→"Maximum Test Number Reached":bool, error out=w1649:errorcluster)  [unwired: 1 in]
        n352 = Variant To Data(error in=w1681, Variant=w1588) -> (data=w1675:bool, error out=w1680:errorcluster)  [unwired: 1 in]
        "Charge FB Fault" <- w1675
        n353 = Variant To Data(error in=w1643, Variant=w1574) -> (data=w1640:bool, error out=w1642:errorcluster)  [unwired: 1 in]
        "Scope Trig" <- w1640
        n354 = Variant To Data(error in=w1755, Variant=w1568) -> (data=w1641:u8, error out=w1711:errorcluster)  [unwired: 1 in]
        "Process Step" <- w1641
        n355 = Variant To Data(error in=w1749, Variant=w1746) -> (data=→"Cap 1 Temperature":i16, error out=w1715:errorcluster)  [unwired: 1 in]
        n356 = Variant To Data(error in=w1748, Variant=w1747) -> (data=w1657:i16, error out=w1713:errorcluster)  [unwired: 1 in]
        "Cap 1 Voltage" <- w1657
        n357 = Variant To Data(error in=w1658, Variant=w1576) -> (data=w1647:i16, error out=w1648:errorcluster)  [unwired: 1 in]
        "Expected Voltage" <- w1647
        n358 = Variant To Data(error in=w1779, Variant=w1778) -> (data=→"Estimated Charge Time (seconds)":sgl, error out=w1707:errorcluster)  [unwired: 1 in]
        n359 = To Double Precision Float(number=w1657) -> (double precision float=→"Waveform Chart - Capacitor Voltage (Probe, abs(Volts))":dbl)
        n360 = Variant To Data(error in=w1758, Variant=w1777) -> (data=→"Shot Number":i16, error out=w1709:errorcluster)  [unwired: 1 in]
        n361 = case shown="True" "Log Temperature Data" {
          tunnel: [errorcluster {"status"=FALSE, "code"=0, "source"=""} ("error out") w1806] -> w1699
          frame False {
          }
          frame True {
            n362 = local read "Cap 1 Temperature"() -> (w1807:i16)
            n363 = local read "test Running"() -> (w1805:bool)
            n364 = call "Write To Measurement File2"("Signals"=w1807, "Enable"=w1805, "Filename"="Capacitor Temperature Data Log File Path (.xlsx)") -> ("error out"=w1806:errorcluster)  [unwired: 14 in, 2 out]
          }
        }
        n365 = case shown="2" w1641 {
          tunnel: ["Charge" "Current Controlled Charge" "Hold - Ready for Shot" "Hold - Cap Open Circuited" "Shot" "Wait" "Dump" "Error" "Wait"] -> w1754
          tunnel: [TRUE TRUE TRUE TRUE TRUE TRUE FALSE FALSE FALSE] -> w1637
          tunnel: [FALSE ("Reset") FALSE ("Reset") FALSE ("Reset") FALSE ("Reset") TRUE ("Reset") FALSE ("Reset") FALSE ("Reset") TRUE ("Reset") FALSE ("Reset")] -> _
          frame 1 {
          }
          frame 6 {
          }
          frame 2 {
          }
          frame 7 {
          }
          frame 3 {
          }
          frame 4 {
          }
          frame 5 {
          }
          frame 99 {
          }
          frame 0, Default {
          }
        }
        "Test State" <- w1754
        n366 = local write "Scope Trig"(w1640) -> ()
        n367 = local read "Cap 1 Voltage"() -> (w1629:i16)
        n368 = case shown="True" "Log Capacitor Voltage" {
          tunnel: [errorcluster {"status"=FALSE, "code"=0, "source"=""} ("error out") w1803] -> w1697
          tunnel: w1657 -> [_ w1802]
          tunnel: w1637 -> [_ w1801]
          frame False {
          }
          frame True {
            n369 = local read "test Running"() -> (w1798:bool)
            n370 = And(x=w1801, y=w1798) -> (x .and. y?=w1799:bool)
            n371 = call "Write To Measurement File"("Signals"=w1802, "Enable"=w1799, "Filename"="Capacitor Voltage Data Log File Path (.xlsx)") -> ("error out"=w1803:errorcluster)  [unwired: 14 in, 2 out]
          }
        }
        n372 = Not(x=w1567) -> (.not. x?=w1655:bool)
        n373 = To Double Precision Float(number=w1629) -> (double precision float=w1653:dbl)
        n374 = To Double Precision Float(number=w1647) -> (double precision float=w1646:dbl)
        n375 = Boolean To (0,1)(Boolean=w1655) -> (0, 1=→"EOC":i16)
        n376 = Or(x=w1732, y=w1733) -> (x .or. y?=w1731:bool)
        n377 = Or(x=w1730, y=w1731) -> (x .or. y?=w1729:bool)
        n378 = Or(x=w1728, y=w1729) -> (x .or. y?=w1727:bool)
        n379 = Or(x=w1726, y=w1727) -> (x .or. y?=w1725:bool)
        n380 = Or(x=w1724, y=w1725) -> (x .or. y?=w1723:bool)
        n381 = Or(x=w1722, y=w1723) -> (x .or. y?=w1721:bool)
        n382 = Or(x=w1720, y=w1721) -> (x .or. y?=w1719:bool)
        n383 = Or(x=w1718, y=w1719) -> (x .or. y?=w1717:bool)
        n384 = Or(x=w1716, y=w1717) -> (x .or. y?=w1704:bool)
        n385 = Or(x=w1705, y=w1704) -> (x .or. y?=w1698:bool)
        n386 = Boolean To (0,1)(Boolean=w1639) -> (0, 1=→"SCR FB":i16)
        n387 = Bundle(w1653, w1646) -> (→"Capacitor Voltage":cluster{dbl, dbl})  [unwired: 1 in]
        n388 = local write "Process Step"(w1641) -> ()
        n389 = local read "Scope Trig"() -> (w1632:bool)
        n390 = local read "Test Interval (Sec)"() -> (w1635:i32)
        n391 = Not(x=w1632) -> (.not. x?=w1631:bool)
        n392 = call "Elapsed Time"("Time Target (s)"=w1635, "Reset"=w1631) -> ("Elapsed Time Text"=w1634:string)  [unwired: 10 in, 7 out]
        n393 = String Subset(string=w1634, offset (0)=2) -> (substring=→"Time Since Last Shot":string)  [unwired: 1 in]
        n394 = Or(x=w1699, y=w1698) -> (x .or. y?=w1696:bool)
        n395 = Or(x=w1697, y=w1696) -> (x .or. y?=w1695:bool)
        n396 = Or(x=w1715, y=w1695) -> (x .or. y?=w1714:bool)
        n397 = Or(x=w1713, y=w1714) -> (x .or. y?=w1712:bool)
        n398 = Or(x=w1711, y=w1712) -> (x .or. y?=w1710:bool)
        n399 = Or(x=w1709, y=w1710) -> (x .or. y?=w1708:bool)
        n400 = Or(x=w1707, y=w1708) -> (x .or. y?=w1706:bool)
        n401 = case shown="True" w1567 {
          frame False {
          }
          frame True {
            n402 = local write "Single"(TRUE) -> ()
          }
        }
        "Internal TwinCAT Handle ID Maps" <- w1616
      }
    }
    n403 = call-poly <userlib>:"Write TypeResolved.vi"("Handle"=w438, "SymbolName"=w510, "WData"=w506, "error constant"=w487) -> ("Write Status?"=w479:bool, "Has Matched?"=w482:bool, "error out"=w504:errorcluster)  [unwired: 8 in, 1 out]
    n404 = call-poly <userlib>:"Write TypeResolved.vi"("Handle"=w438, "SymbolName"=w511, "WData"=w507, "error constant"=w487) -> ("Write Status?"=w478:bool, "Has Matched?"=w483:bool, "error out"=w505:errorcluster)  [unwired: 8 in, 1 out]
    n405 = call <userlib>:"Send Writer-Request.vi"("Handle"=w970, "SymbolName"=w969, "WriterMode"=w968, "WriteHandle"=w967, "error constant"=w966, "ADS Write Data"=w721) -> ("Handle"=w962:u32, "WriteHandle"=w961:u32, "Write status?"=w699:bool, "error IO"=w654:errorcluster)  [unwired: 5 in, 1 out]
    n406 = call-poly <userlib>:"Write TypeResolved.vi"("Handle"=w438, "SymbolName"=w525, "WData"=w519, "error constant"=w524) -> ("Handle"=w520:u32, "Write Status?"=w477:bool, "Has Matched?"=w485:bool, "error out"=w521:errorcluster)  [unwired: 8 in]
    n407 = call <userlib>:"Send Writer-Request.vi"("Handle"=w886, "SymbolName"=w885, "WriterMode"=w884, "WriteHandle"=w882, "error constant"=w883, "ADS Write Data"=w805) -> ("Handle"=w881:u32, "WriteHandle"=w880:u32, "Write status?"=w501:bool, "error IO"=w634:errorcluster)  [unwired: 5 in, 1 out]
    n408 = call <userlib>:"Send Writer-Request.vi"("Handle"=w796, "SymbolName"=w795, "WriterMode"=w794, "WriteHandle"=w785, "error constant"=w793, "ADS Write Data"=w465) -> ("Handle"=w792:u32, "WriteHandle"=w791:u32, "Write status?"=w496:bool, "error IO"=w464:errorcluster)  [unwired: 5 in, 1 out]
    n409 = call <userlib>:"Send Writer-Request.vi"("Handle"=w874, "SymbolName"=w873, "WriterMode"=w872, "WriteHandle"=w871, "error constant"=w870, "ADS Write Data"=w804) -> ("Handle"=w866:u32, "WriteHandle"=w865:u32, "Write status?"=w500:bool, "error IO"=w631:errorcluster)  [unwired: 5 in, 1 out]
    n410 = call <userlib>:"Send Writer-Request.vi"("Handle"=w850, "SymbolName"=w849, "WriterMode"=w848, "WriteHandle"=w847, "error constant"=w846, "ADS Write Data"=w802) -> ("Handle"=w842:u32, "WriteHandle"=w841:u32, "Write status?"=w498:bool, "error IO"=w625:errorcluster)  [unwired: 5 in, 1 out]
    n411 = call <userlib>:"Send Writer-Request.vi"("Handle"=w862, "SymbolName"=w861, "WriterMode"=w860, "WriteHandle"=w859, "error constant"=w858, "ADS Write Data"=w803) -> ("Handle"=w854:u32, "WriteHandle"=w853:u32, "Write status?"=w499:bool, "error IO"=w628:errorcluster)  [unwired: 5 in, 1 out]
    n412 = call <userlib>:"Send Writer-Request.vi"("Handle"=w838, "SymbolName"=w837, "WriterMode"=w836, "WriteHandle"=w835, "error constant"=w834, "ADS Write Data"=w801) -> ("Handle"=w830:u32, "WriteHandle"=w829:u32, "Write status?"=w497:bool, "error IO"=w622:errorcluster)  [unwired: 5 in, 1 out]
    n413 = call <userlib>:"Send Writer-Request.vi"("Handle"=w958, "SymbolName"=w957, "WriterMode"=w956, "WriteHandle"=w954, "error constant"=w955, "ADS Write Data"=w811) -> ("Handle"=w953:u32, "WriteHandle"=w952:u32, "Write status?"=w687:bool, "error IO"=w651:errorcluster)  [unwired: 5 in, 1 out]
    n414 = call <userlib>:"Send Writer-Request.vi"("Handle"=w898, "SymbolName"=w897, "WriterMode"=w896, "WriteHandle"=w895, "error constant"=w894, "ADS Write Data"=w806) -> ("Handle"=w890:u32, "WriteHandle"=w889:u32, "Write status?"=w697:bool, "error IO"=w636:errorcluster)  [unwired: 5 in, 1 out]
    n415 = call <userlib>:"Send Writer-Request.vi"("Handle"=w946, "SymbolName"=w945, "WriterMode"=w944, "WriteHandle"=w943, "error constant"=w942, "ADS Write Data"=w810) -> ("Handle"=w938:u32, "WriteHandle"=w937:u32, "Write status?"=w689:bool, "error IO"=w648:errorcluster)  [unwired: 5 in, 1 out]
    n416 = call <userlib>:"Send Writer-Request.vi"("Handle"=w922, "SymbolName"=w921, "WriterMode"=w920, "WriteHandle"=w919, "error constant"=w918, "ADS Write Data"=w808) -> ("Handle"=w914:u32, "WriteHandle"=w913:u32, "Write status?"=w693:bool, "error IO"=w642:errorcluster)  [unwired: 5 in, 1 out]
    n417 = call <userlib>:"Send Writer-Request.vi"("Handle"=w934, "SymbolName"=w933, "WriterMode"=w932, "WriteHandle"=w931, "error constant"=w930, "ADS Write Data"=w809) -> ("Handle"=w926:u32, "WriteHandle"=w925:u32, "Write status?"=w691:bool, "error IO"=w645:errorcluster)  [unwired: 5 in, 1 out]
    n418 = call <userlib>:"Send Writer-Request.vi"("Handle"=w910, "SymbolName"=w909, "WriterMode"=w908, "WriteHandle"=w907, "error constant"=w906, "ADS Write Data"=w807) -> ("Handle"=w902:u32, "WriteHandle"=w901:u32, "Write status?"=w695:bool, "error IO"=w639:errorcluster)  [unwired: 5 in, 1 out]
    n419 = call <userlib>:"Send Writer-Request.vi"("Handle"=w614, "SymbolName"=w613, "WriterMode"=w612, "WriteHandle"=w611, "error constant"=w610, "ADS Write Data"=w606) -> ("Handle"=w605:u32, "WriteHandle"=w604:u32, "Write status?"=w598:bool, "error IO"=w461:errorcluster)  [unwired: 5 in, 1 out]
    n420 = Compound Arithmetic op=AND(w485, w483, w482, w481) -> (w484:bool)
    n421 = And(x=w454, y=w484) -> (x .and. y?=w522:bool)
    n422 = And(x=w444, y=w522) -> (x .and. y?=w596:bool)
    n423 = And(x=w683, y=w596) -> (x .and. y?=w682:bool)
    n424 = And(x=w434, y=w682) -> (x .and. y?=w681:bool)
    n425 = And(x=w680, y=w681) -> (x .and. y?=w679:bool)
    n426 = And(x=w678, y=w679) -> (x .and. y?=w677:bool)
    n427 = And(x=w676, y=w677) -> (x .and. y?=w675:bool)
    n428 = And(x=w674, y=w675) -> (x .and. y?=w673:bool)
    n429 = And(x=w672, y=w673) -> (x .and. y?=w589:bool)
    n430 = And(x=w600, y=w589) -> (x .and. y?=w601:bool)
    n431 = And(x=w671, y=w601) -> (x .and. y?=w670:bool)
    n432 = And(x=w669, y=w670) -> (x .and. y?=w668:bool)
    n433 = And(x=w667, y=w668) -> (x .and. y?=w666:bool)
    n434 = And(x=w665, y=w666) -> (x .and. y?=w664:bool)
    n435 = And(x=w663, y=w664) -> (x .and. y?=w662:bool)
    n436 = And(x=w661, y=w662) -> (x .and. y?=w660:bool)
    n437 = And(x=w659, y=w660) -> (x .and. y?=w658:bool)
    n438 = And(x=w685, y=w658) -> (x .and. y?=→"bHasMached":bool)
    n439 = Compound Arithmetic op=AND(w477, w478, w479, w480) -> (w476:bool)
    n440 = And(x=w452, y=w476) -> (x .and. y?=w523:bool)
    n441 = And(x=w443, y=w523) -> (x .and. y?=w493:bool)
    n442 = Compound Arithmetic op=AND(w501, w500, w499, w498, w497, w433, w496) -> (w495:bool)
    n443 = Not(x=w495) -> (.not. x?=w494:bool)
    n444 = And(x=w494, y=w493) -> (x .and. y?=w492:bool)
    n445 = And(x=w598, y=w492) -> (x .and. y?=w599:bool)
    n446 = And(x=w697, y=w599) -> (x .and. y?=w696:bool)
    n447 = And(x=w695, y=w696) -> (x .and. y?=w694:bool)
    n448 = And(x=w693, y=w694) -> (x .and. y?=w692:bool)
    n449 = And(x=w691, y=w692) -> (x .and. y?=w690:bool)
    n450 = And(x=w689, y=w690) -> (x .and. y?=w688:bool)
    n451 = And(x=w687, y=w688) -> (x .and. y?=w686:bool)
    n452 = And(x=w699, y=w686) -> (x .and. y?=w698:bool)
    n453 = And(x=w700, y=w698) -> (x .and. y?=→"Write Status":bool)
    n454 = feedback #2(TRUE) -> (w545:bool)
    n455 = And(x=w545, y=w548) -> (x .and. y?=w547:bool)
    n456 = feedback #3(TRUE) -> (w555:bool)
    n457 = And(x=w555, y=w558) -> (x .and. y?=w557:bool)
    n458 = feedback #4(TRUE) -> (w559:bool)
    n459 = And(x=w559, y=w562) -> (x .and. y?=w561:bool)
    n460 = feedback #5(TRUE) -> (w551:bool)
    n461 = And(x=w551, y=w550) -> (x .and. y?=w552:bool)
    n462 = case shown="True" w552 {
      tunnel: [w1165 FALSE] -> w542
      tunnel: w543 -> [w1167 _]
      frame False {
        n463 = Or(x=w1167, y=FALSE) -> (x .or. y?=w1165:bool)
      }
      frame True {
        n464 = call "Charge relay error"() -> ()  [unwired: 10 in, 2 out]
      }
    }
    n465 = feedback-in #5(w542) -> ()
    n466 = case shown="True" w547 {
      tunnel: [w1163 FALSE] -> w546
      tunnel: w542 -> [w1161 _]
      frame False {
        n467 = Or(x=w1161, y=FALSE) -> (x .or. y?=w1163:bool)
      }
      frame True {
        n468 = call "PSU HV error"() -> ()  [unwired: 10 in, 2 out]
      }
    }
    n469 = feedback-in #2(w546) -> ()
    n470 = case shown="True" w561 {
      tunnel: [w1174 FALSE] -> w560
      tunnel: w543 -> [w1173 _]
      frame False {
        n471 = Or(x=w1173, y=FALSE) -> (x .or. y?=w1174:bool)
      }
      frame True {
        n472 = call "Softdump error"() -> ()  [unwired: 10 in, 2 out]
      }
    }
    n473 = feedback-in #4(w560) -> ()
    n474 = case shown="True" w557 {
      tunnel: [w1169 FALSE] -> w556
      tunnel: w542 -> [w1170 _]
      frame False {
        n475 = Or(x=w1170, y=FALSE) -> (x .or. y?=w1169:bool)
      }
      frame True {
        n476 = call "Soft Exception"() -> ()  [unwired: 10 in, 2 out]
      }
    }
    n477 = feedback-in #3(w556) -> ()
    n478 = Compound Arithmetic op=OR(w620, w657, w656) -> (w655:bool)
    n479 = Compound Arithmetic op=OR(w655, w654, w653) -> (w652:bool)
    n480 = Compound Arithmetic op=OR(w652, w651, w650) -> (w649:bool)
    n481 = Compound Arithmetic op=OR(w649, w648, w647) -> (w646:bool)
    n482 = Compound Arithmetic op=OR(w646, w645, w644) -> (w643:bool)
    n483 = Compound Arithmetic op=OR(w643, w642, w641) -> (w640:bool)
    n484 = Compound Arithmetic op=OR(w640, w639, w638) -> (w637:bool)
    n485 = Compound Arithmetic op=OR(w637, w636, w635) -> (w597:bool)
    n486 = Compound Arithmetic op=OR(w597, w461, w460) -> (w588:bool)
    n487 = Compound Arithmetic op=OR(w588, w634, w633) -> (w632:bool)
    n488 = Compound Arithmetic op=OR(w632, w631, w630) -> (w629:bool)
    n489 = Compound Arithmetic op=OR(w629, w628, w627) -> (w626:bool)
    n490 = Compound Arithmetic op=OR(w626, w625, w624) -> (w623:bool)
    n491 = Compound Arithmetic op=OR(w623, w622, w621) -> (w435:bool)
    n492 = Compound Arithmetic op=OR(w435, w464, w463) -> (w445:bool)
    n493 = Compound Arithmetic op=OR(w445, "EXIT HMI", w432) -> (w431:bool)
    "Stop Loops" <- w431
    n494 = property on="Stop Loops" class="Bool (strict)"("Val(Sgnl)"=w431) -> ()  [unwired: 2 in, 2 out]
    n495 = node-c288() -> ()  [unwired: 1 in, 1 out]
  }
  n496 = node-c288(w95) -> (w94:errorcluster)
  n497 = call <userlib>:"Release Writer.vi"("Handle"=w265, "WriteHandle"=w264, "error in (no error)"=w263) -> ("error out"=w271:errorcluster)  [unwired: 11 in, 1 out]
  n498 = call <userlib>:"Release Writer.vi"("Handle"=w245, "WriteHandle"=w244, "error in (no error)"=w243) -> ("error out"=w239:errorcluster)  [unwired: 11 in, 1 out]
  n499 = call <userlib>:"Release Writer.vi"("Handle"=w207, "WriteHandle"=w206, "error in (no error)"=w205) -> ("error out"=w201:errorcluster)  [unwired: 11 in, 1 out]
  n500 = call <userlib>:"Release Type.vi"("Handle"=w260, "TypeHandle"=w261, "error in (no error)"=w262) -> ("error out"=w272:errorcluster)  [unwired: 11 in, 1 out]
  n501 = call <userlib>:"Release Type.vi"("Handle"=w242, "TypeHandle"=w241, "error in (no error)"=w240) -> ("error out"=w238:errorcluster)  [unwired: 11 in, 1 out]
  n502 = call <userlib>:"Release Writer.vi"("Handle"=w226, "WriteHandle"=w225, "error in (no error)"=w224) -> ("error out"=w220:errorcluster)  [unwired: 11 in, 1 out]
  n503 = call <userlib>:"Release Type.vi"("Handle"=w204, "TypeHandle"=w203, "error in (no error)"=w202) -> ("error out"=w200:errorcluster)  [unwired: 11 in, 1 out]
  n504 = call <userlib>:"Release Writer.vi"("Handle"=w188, "WriteHandle"=w187, "error in (no error)"=w186) -> ("error out"=w182:errorcluster)  [unwired: 11 in, 1 out]
  n505 = call <userlib>:"Release Type.vi"("Handle"=w223, "TypeHandle"=w222, "error in (no error)"=w221) -> ("error out"=w219:errorcluster)  [unwired: 11 in, 1 out]
  n506 = call <userlib>:"Release Type.vi"("Handle"=w185, "TypeHandle"=w184, "error in (no error)"=w183) -> ("error out"=w181:errorcluster)  [unwired: 11 in, 1 out]
  n507 = call <userlib>:"Release Writer.vi"("Handle"=w414, "WriteHandle"=w413, "error in (no error)"=w424) -> ("error out"=w114:errorcluster)  [unwired: 11 in, 1 out]
  n508 = call <userlib>:"Release Writer.vi"("Handle"=w283, "WriteHandle"=w282, "error in (no error)"=w281) -> ("error out"=w277:errorcluster)  [unwired: 11 in, 1 out]
  n509 = call <userlib>:"Release Writer.vi"("Handle"=w379, "WriteHandle"=w378, "error in (no error)"=w377) -> ("error out"=w385:errorcluster)  [unwired: 11 in, 1 out]
  n510 = call <userlib>:"Release Writer.vi"("Handle"=w359, "WriteHandle"=w358, "error in (no error)"=w357) -> ("error out"=w353:errorcluster)  [unwired: 11 in, 1 out]
  n511 = call <userlib>:"Release Writer.vi"("Handle"=w321, "WriteHandle"=w320, "error in (no error)"=w319) -> ("error out"=w315:errorcluster)  [unwired: 11 in, 1 out]
  n512 = call <userlib>:"Release Type.vi"("Handle"=w280, "TypeHandle"=w279, "error in (no error)"=w278) -> ("error out"=w276:errorcluster)  [unwired: 11 in, 1 out]
  n513 = call <userlib>:"Release Type.vi"("Handle"=w374, "TypeHandle"=w375, "error in (no error)"=w376) -> ("error out"=w386:errorcluster)  [unwired: 11 in, 1 out]
  n514 = call <userlib>:"Release Type.vi"("Handle"=w356, "TypeHandle"=w355, "error in (no error)"=w354) -> ("error out"=w352:errorcluster)  [unwired: 11 in, 1 out]
  n515 = call <userlib>:"Release Writer.vi"("Handle"=w340, "WriteHandle"=w339, "error in (no error)"=w338) -> ("error out"=w334:errorcluster)  [unwired: 11 in, 1 out]
  n516 = call <userlib>:"Release Type.vi"("Handle"=w318, "TypeHandle"=w317, "error in (no error)"=w316) -> ("error out"=w314:errorcluster)  [unwired: 11 in, 1 out]
  n517 = call <userlib>:"Release Writer.vi"("Handle"=w302, "WriteHandle"=w301, "error in (no error)"=w300) -> ("error out"=w296:errorcluster)  [unwired: 11 in, 1 out]
  n518 = call <userlib>:"Release Type.vi"("Handle"=w337, "TypeHandle"=w336, "error in (no error)"=w335) -> ("error out"=w333:errorcluster)  [unwired: 11 in, 1 out]
  n519 = call <userlib>:"Release Type.vi"("Handle"=w299, "TypeHandle"=w298, "error in (no error)"=w297) -> ("error out"=w295:errorcluster)  [unwired: 11 in, 1 out]
  n520 = call <userlib>:"Release Writer.vi"("Handle"=w397, "WriteHandle"=w396, "error in (no error)"=w395) -> ("error out"=w391:errorcluster)  [unwired: 11 in, 1 out]
  n521 = call <userlib>:"Release Writer.vi"("Handle"=w78, "WriteHandle"=w77, "error in (no error)"=w10) -> ("error out"=w92:errorcluster)  [unwired: 11 in, 1 out]
  n522 = call <userlib>:"Release Writer.vi"("Handle"=w12, "WriteHandle"=w150, "error in (no error)"=w15) -> ("Handle"=w4:u32, "error out"=w156:errorcluster)  [unwired: 11 in]
  n523 = call <userlib>:"Release Type.vi"("Handle"=w394, "TypeHandle"=w393, "error in (no error)"=w392) -> ("error out"=w390:errorcluster)  [unwired: 11 in, 1 out]
  n524 = call <userlib>:"Release Type.vi"("Handle"=w76, "TypeHandle"=w75, "error in (no error)"=w9) -> ("error out"=w91:errorcluster)  [unwired: 11 in, 1 out]
  n525 = call <userlib>:"Release Type.vi"("Handle"=w146, "TypeHandle"=w145, "error in (no error)"=w14) -> ("error out"=w155:errorcluster)  [unwired: 11 in, 1 out]
  n526 = call <userlib>:"Release Type.vi"("Handle"=w412, "TypeHandle"=w411, "error in (no error)"=w423) -> ("error out"=w115:errorcluster)  [unwired: 11 in, 1 out]
  n527 = Merge Errors(w271, w272) -> (w103:errorcluster)
  n528 = Merge Errors(w239, w238) -> (w102:errorcluster)
  n529 = Merge Errors(w201, w200) -> (w100:errorcluster)
  n530 = Merge Errors(w220, w219) -> (w101:errorcluster)
  n531 = Merge Errors(w182, w181) -> (w99:errorcluster)
  n532 = Merge Errors(w385, w386) -> (w109:errorcluster)
  n533 = Merge Errors(w277, w276) -> (w104:errorcluster)
  n534 = Merge Errors(w353, w352) -> (w108:errorcluster)
  n535 = Merge Errors(w315, w314) -> (w106:errorcluster)
  n536 = Merge Errors(w334, w333) -> (w107:errorcluster)
  n537 = Merge Errors(w296, w295) -> (w105:errorcluster)
  n538 = Merge Errors(w391, w390) -> (w110:errorcluster)
  n539 = Merge Errors(w92, w91) -> (w90:errorcluster)
  n540 = Merge Errors(w156, w155) -> (w98:errorcluster)
  n541 = Merge Errors(w114, w115) -> (w113:errorcluster)
  n542 = Merge Errors(w46, w45, w44, w43, w35, w17, w16) -> (w41:errorcluster)
  n543 = Merge Errors(w109, w108, w107, w106, w105, w104, w90) -> (w173:errorcluster)
  n544 = Merge Errors(w103, w102, w101, w100, w99, w1, w98, w5, w7, w30, w29, w28, w24) -> (w172:errorcluster)
  n545 = Merge Errors(w125, w126, w127, w128, w129, w71, w70, w66, w67, w68, w69) -> (w116:errorcluster)
  n546 = Merge Errors(w93, w124, w123, w122, w121, w120, w119, w118, w57, w56, w55, w42, w41) -> (w117:errorcluster)
  n547 = Merge Errors(w116, w117) -> (w23:errorcluster)
  n548 = Merge Errors(w94, w113, w110, w173, w172, w23) -> (w111:errorcluster)
  n549 = call <userlib>:"Release.vi"("Handle"=w4, "error in (no error)"=w111) -> ("error out"=→"error out":errorcluster)  [unwired: 13 in]
